vi "MDO-Monitor main_design.vi"() -> ()   [LabVIEW 2012]
uses:
  SubVI/Controls/main_states.ctl
  SubVI/Controls/options.ctl
  SubVI/Controls/Globol_Data_Cluster.ctl
  SubVI/Controls/main_tab.ctl
  SubVI/Controls/process condition.ctl
  SubVI/Controls/MBA_data.ctl
  <vilib>/Utility/miscctls.llb/LVRowAndColumnTypeDef.ctl
  <vilib>/Utility/error.llb/DialogType.ctl
  <vilib>/Utility/file.llb/Write To Spreadsheet File (string).vi
  <vilib>/Analysis/5stat.llb/RMS (DBL).vi
  <vilib>/Analysis/baseanly.llb/Mean (DBL).vi
  <vilib>/Analysis/NI_AALPro.lvlib
  <vilib>/Analysis/NI_AALBase.lvlib
panel:
  out "Sreaming_Execution:State":T1(ring)
  out "Application Directory":path
  out "Max_voltage":dbl
  out "states_history":string
  out "current_state":T2
  out "Main Tab":T3(tab)
  in  "stop":bool
  in  "МДО-Настройщик":bool
  in  "МДО-Монитор":bool
  out "current time":timestamp format="%<%X\n%x>T"
  in  "МДО-Принтер":bool
  in  "МДО-Визуализатор":bool
  in  "Electrolyte composition":string[][](table)=[["KOH", "2"], ["Жидкое стекло", "9"]] caption="Состав электролита"
  in  "Дата проведения процесса":string
  in  "Время проведения процесса":string
  in  "Предмет исследований":string
  in  "Сплав":string
  in  "Очистить все поля":bool
  out "Ti литейные сплавы":string="Ti литейный"
  out "Ti деформируемые сплавы":string="Ti деформ"
  out "Mg литейные сплавы":string="Mg литейный"
  out "Mg деформируемые сплавы":string="Mg деформ"
  out "Al деформируемые сплавы":string="Al деформ"
  out "Al литейные сплавы":string="Al литейный"
  out "Список сплавов":string[][](table)
  in  "MDO_mode":string(combo)="ПОЭП"
  in  "Bath volume":string(combo)="800 л"
  in  "MDO duration":i32
  in  "К процессу":bool
  in  "Пауза":bool
  in  "Принудительный запуск":bool
  in  "Отложенный запуск":bool
  in  "СТОП":bool
  in  "Graph Tab":T4(tab)
  out "Катодный ток, А":cluster{dbl, dbl, dbl}(knob) scale=0.0..40.0
  out "Анодный ток, А":cluster{dbl, dbl, dbl}(knob) scale=0.0..40.0 scale format="%#.1g"
  out "Катодное напряжение, В":cluster{u16, u16, u16}(knob) scale=0.0..200.0
  out "Анодное напряжение, В":cluster{u16, u16, u16}(knob) scale=0.0..800.0
  out "XY Graph":cluster{"all rows":dbl[], "all rows":dbl[]}(graph)
  out "Currency":dbl[](graph)
  out "Voltage":dbl[](graph)
  in  "anod/katod_Form":bool
  out "Формовочный ток":cluster{dbl, dbl, dbl}(graph)
  out "Формовочное напряжение":cluster{u16, u16, u16}(graph)
  out "Process Electrical Parameters":string[][](table)
  out "Bath type":string caption="Ванна"
  out "Electrolyte temperature":dbl(slide) caption="Температура электролита" scale=0.0..60.0
  out "Cooler flow":dbl(knob) caption="Давление воды в системе охлаждения" scale=0.0..3.5 scale format="%#_2g"
  out "Bubbling flow":bool caption="Расход газа в барботере"
  out "Ventilation flow":bool caption="Расход газа в вытяжке"
  in  "ВЫХОД":bool
  in  "НОВЫЙ СБОР":bool
  out "ДАННЫЕ СОХРАНЕНЫ":string="ДАННЫЕ СОХРАНЕНЫ"
  in  "Save_data":bool
  in  "ПРИМЕЧАНИЕ":bool
  in  "ТОК ТОЧНО":u8(slide)=5 max=10 step=1 scale=0.0..10.0
  in  "ТОК ГРУБО":u8(slide)=1 max=2 step=1 scale=0.0..2.0
  in  "ПРЕДЕЛЫ ПО НАПРЯЖ":bool=TRUE
  in  "СТОП - КАДР":bool
  in  "Boolean":bool
  out "ТАЙМЕР Текущий":string
  out "УГАСАНИЕ":string="УГАСАНИЕ"
  out "ДР":string="Д Р"
  out "ИР":string="И Р"
  out "ГАЛЬВ.ЛЮМ.":string="ГАЛЬВ"
  out "МДР":string="МДР"
  out "依商判":string
  out "СТОП":string="СТОП"
  out "ПАУЗА":string="ПАУЗА"
  out "СБОР":string="СБОР"
  out "Готовность":string="ГОТОВ"
  in  "End vizualization":bool
  in  "End print":bool
  in  "Options":T5={"Form_data_log_period"=0, "startup_threshold"=0.0, "Coeff_U"=2.55, "Offset_U"=6.5, "Coeff_I"=42.391, "Offset_I"=77.0, "Save_data_path"=path "", "ADC_frequency"=50000.0, "VISA resource name"="COM1"} caption="Настройки"
  in  "Apply options":bool
  in  "Cancel options":bool
  # "МДО-Монитор"
  # "Мониторинг электрических технологических параметров процесса микродугового оксидирования и обновление базы данных МДО"
  # "МДО-Настройщик"
  # "Настройка параметров \nМДО-Инструментарий"
  # "Пожалуйста, заполните описание эксперимента"
  # "Дата и время проведения процесса"
  # "Цель исследования"
  # "Сплав"
  # "Электролит"
  # "Очистить все поля"
  # "Ванна"
  # "ТИТ"
  # "Длительность"
  # "мин"
  # "ПАНЕЛЬ ЗАПУСКА"
  # "ПУСК СЛЕДЯЩИЙ"
  # "ПУСК ПРИНУДИТ"
  # "ПАУЗА"
  # "СТОП"
  # "АПЛИТУДНЫЙ\nДЕЙСТВУЮЩИЙ\nСРЕДНИЙ"
  # "АПЛИТУДНОЕ\nДЕЙСТВУЮЩЕЕ\nСРЕДНЕЕ"
  # "劳文"
  # "КАТОД"
  # "о"
  # "С"
  # "атм"
  # "ПАНЕЛЬ УПРАВЛЕНИЯ"
  # "ГРУБО"
  # "ТОЧНО"
  # "ПРЕДЕЛЫ"
  # "ПО ТОКУ"
  # "800 /200"
  # "1000 / 250"
  # "ПРЕДЕЛЫ"
  # "ПО НАПРЯЖ"
  # "ПАНЕЛЬ ИНДИКАЦИИ"
  # "Принудительная остановка"
  # "Здесь будет"
  # "Визуализатор"
  # "Визуализация электрических технологических параметров процесса микродугового оксидирования по базе данных МДО"
  # "Здесь будет"
  # "Принтер"
  # "Распечатка графиков электрических параметров процесса МДО (осциллограммы, ВАХи, форовочные кривые) по базе данных МДО"
  # "с"
  # "В"
  # "Настройки АЦП"
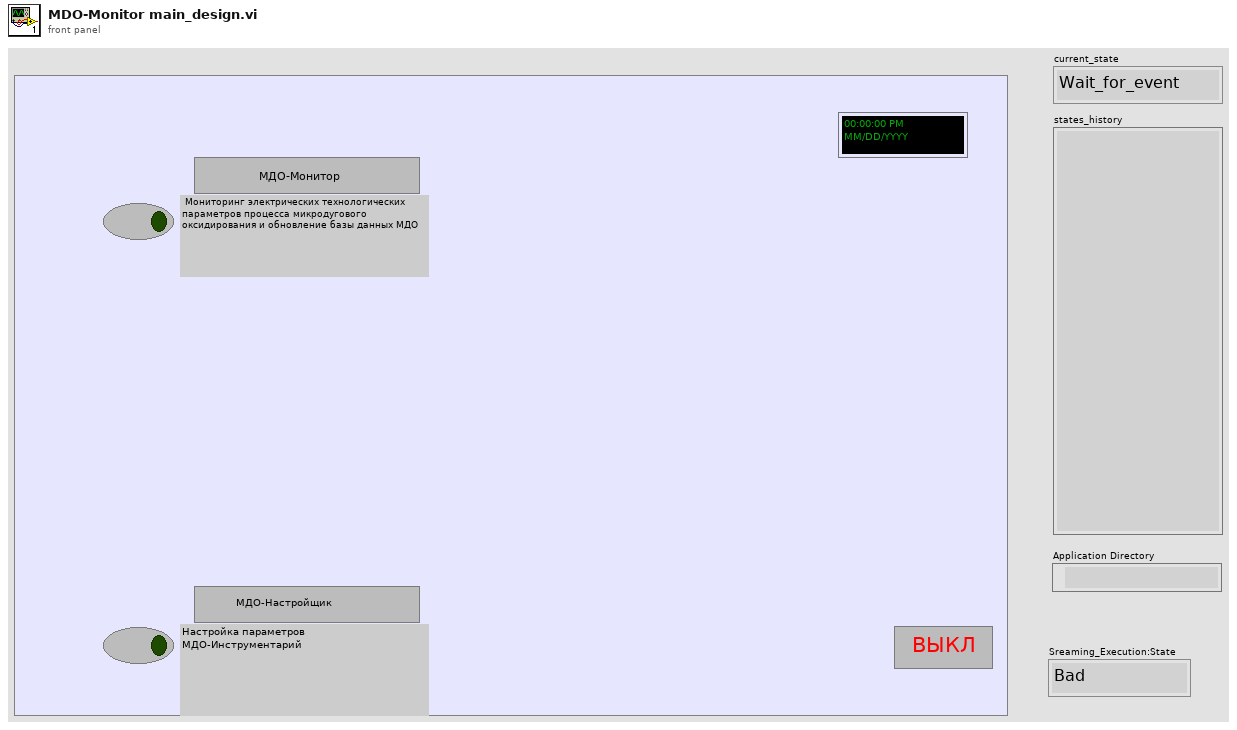
[diagram p1: front panel]
types:
  T1 = enum32{"Bad", "Idle", "Run top level", "Running"}
  T2 = typedef "main_states.ctl" = enum16{"Wait_for_event", "Initialize", "Save_ini", "Save_data", "Streaming_config", "Streaming_open", "Streaming_monitor", "Streaming_stop", "Vizualyze", "Form_data_fetch", "Process_analyze", "Start_data_loging", "Pause_data_loging", "Stop_data_loging", "Reset_data_colection", "Error_handler", "Stop"}
  T3 = enum32{"Выбор", "Описание эксперимента", "Монитор", "Визуализатор", "Принтер", "Настройщик"}
  T4 = enum32{"Осциллограммы/ВАХи", "Формовочные кривые", "Электрические параметры", "Состояние оборудования "}
  T5 = typedef "options.ctl" = cluster{"Form_data_log_period":i32, "startup_threshold":dbl, "Coeff_U":dbl, "Offset_U":dbl, "Coeff_I":dbl, "Offset_I":dbl, "Save_data_path":path, "ADC_frequency":dbl, "VISA resource name":refnum<visa-resource-name>}
  T6 = typedef "Globol_Data_Cluster.ctl" = cluster{"Streaming_enable":bool, "Options":T5, "Ini_file_path":path, "Global_errors":errorcluster, "Main Tab":T7, "Process conditions":T8, "App_directory_path":path, "Data_write_enable":bool, "Process_time":u32, "Current":dbl[], "Voltag":dbl[], "startup_time":u32, "Streaming Refnum":refnum<vi>, "Note Refnum":refnum<vi>, "Note":string, "Modbus spy Refnum":refnum<vi>, "MBA data":T9, "shutdown?":bool, "Oscil_path":path, " Data log path":path}
  T7 = typedef "main_tab.ctl" = enum32{"Выбор", "Описание эксперимента", "Монитор", "Визуализатор", "Принтер", "Настройщик"}
  T8 = typedef "process condition.ctl" = cluster{"Data":string, "Time":string, "Subject":string, "Research target":string, "Material":string, "Electrolyte composition":string[][], "MDO mode":string, "Bath volume":string, "Process duration":i32}
  T9 = typedef "MBA_data.ctl" = cluster{"MBA_ch 1":dbl, "MBA_ch 2":dbl, "MBA_ch 3":dbl, "MBA_ch 4":dbl, "MBA_ch 5":dbl, "MBA_ch 6":dbl, "MBA_ch 7":dbl, "MBA_ch 8":dbl}
  T10 = typedef "LVRowAndColumnTypeDef.ctl" = cluster{"Row":i32, "Column":i32}
  T11 = enum16{"open", "replace", "create", "open or create", "replace or create", "replace or create with confirmation"}
  T12 = enum32{"invalid app kind", "Development System", "Run Time System", "Student Edition", "Embedded LabVIEW", "Evaluation", "Custom"}
  T13 = typedef "DialogType.ctl" = u16
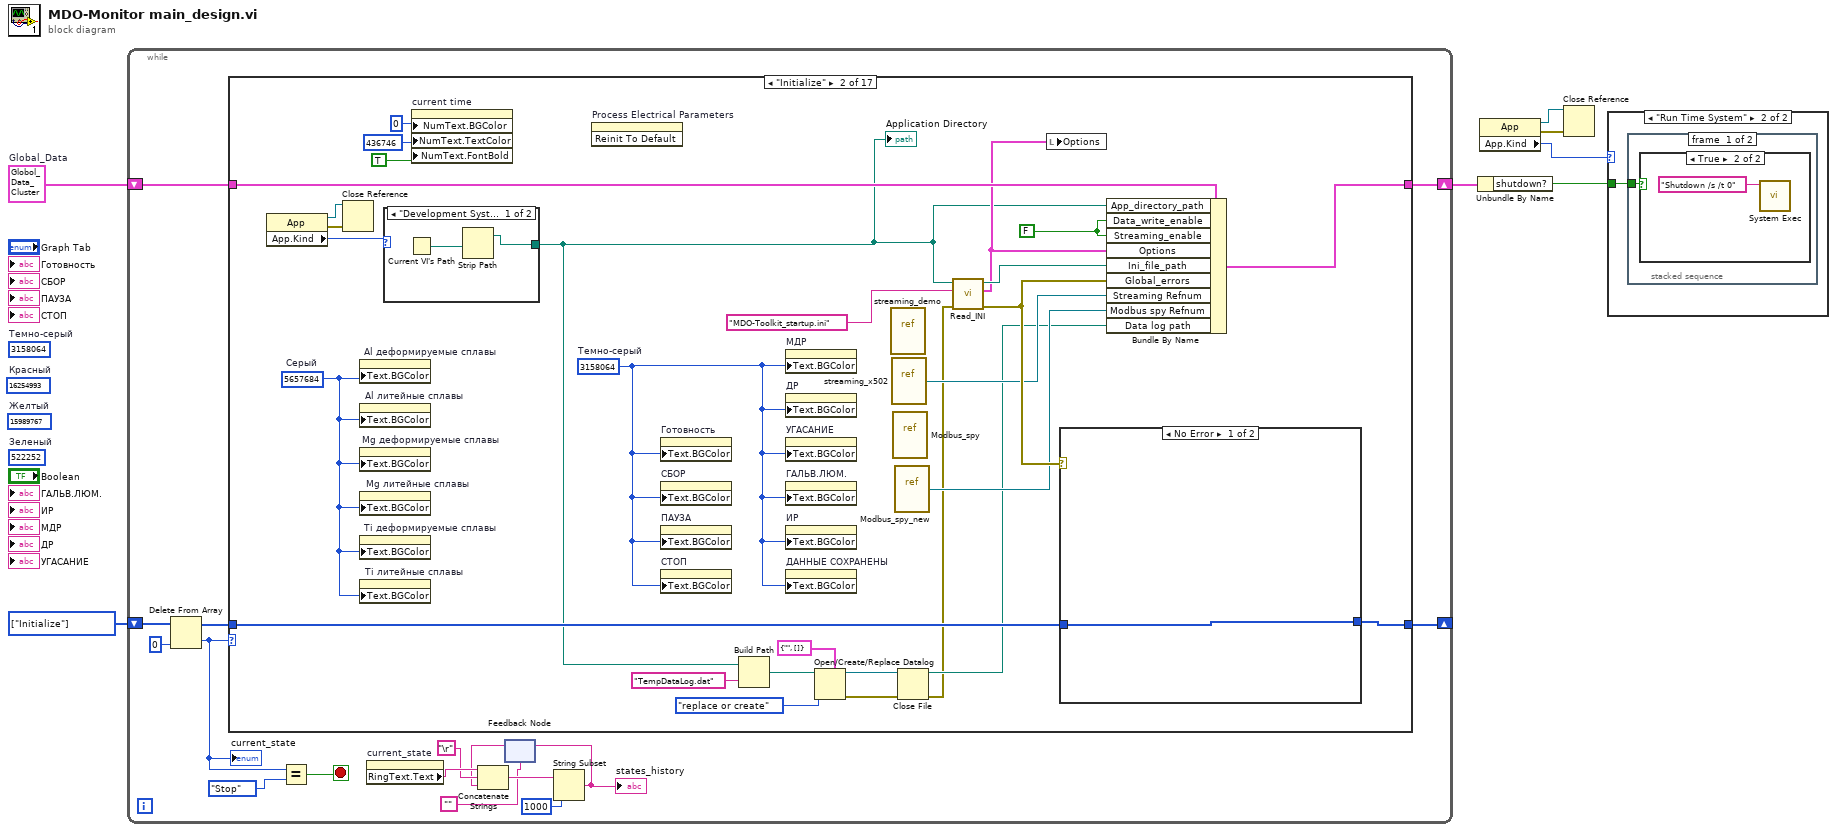
[diagram p0: block diagram]
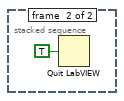
[diagram p4: hidden frame]
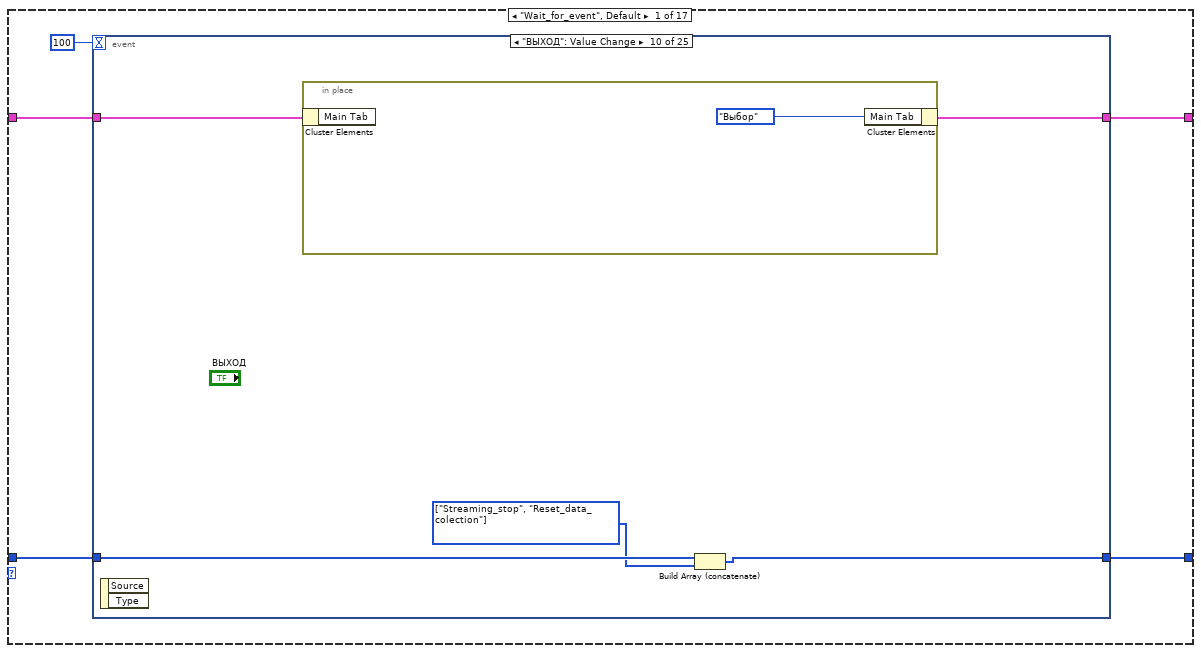
[diagram p5: hidden frame]
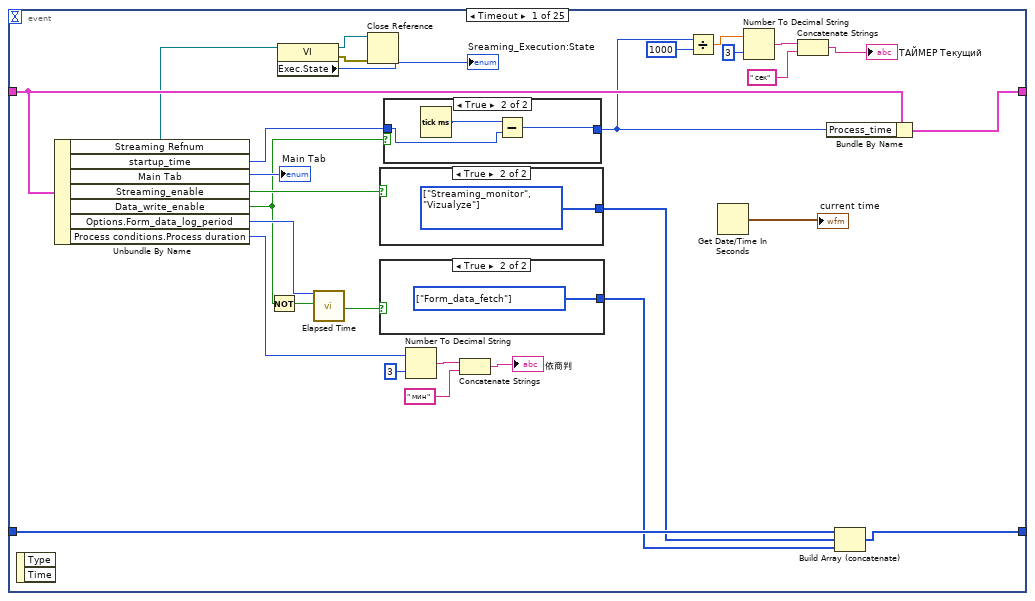
[diagram p6: hidden frame]
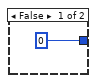
[diagram p7: hidden frame]
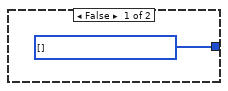
[diagram p8: hidden frame]
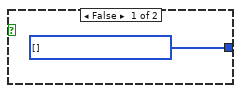
[diagram p9: hidden frame]
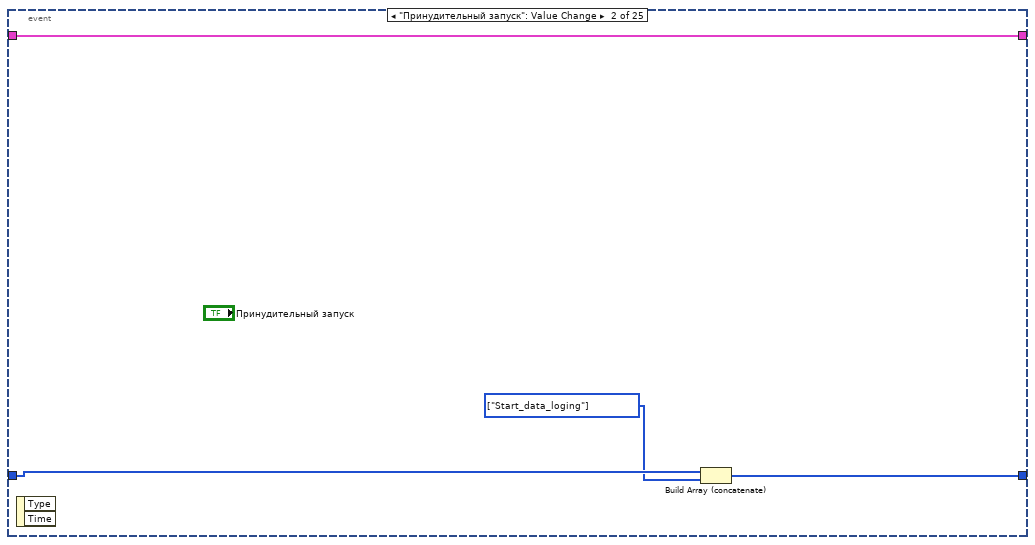
[diagram p10: hidden frame]
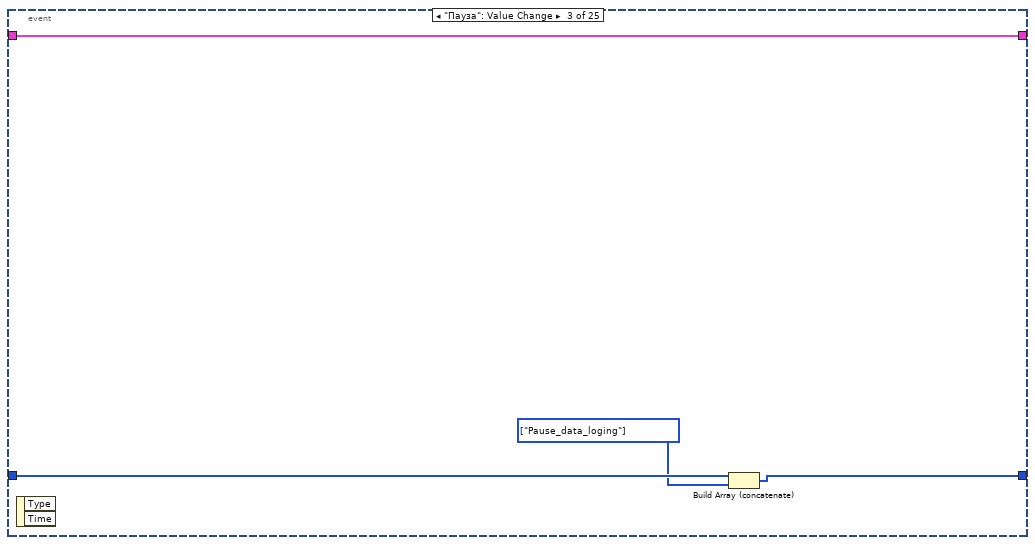
[diagram p11: hidden frame]
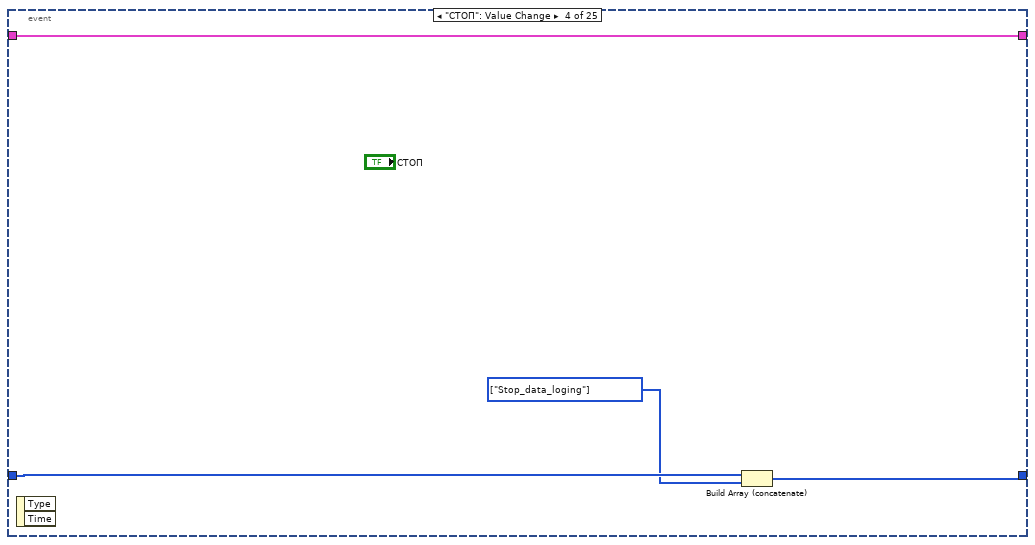
[diagram p12: hidden frame]
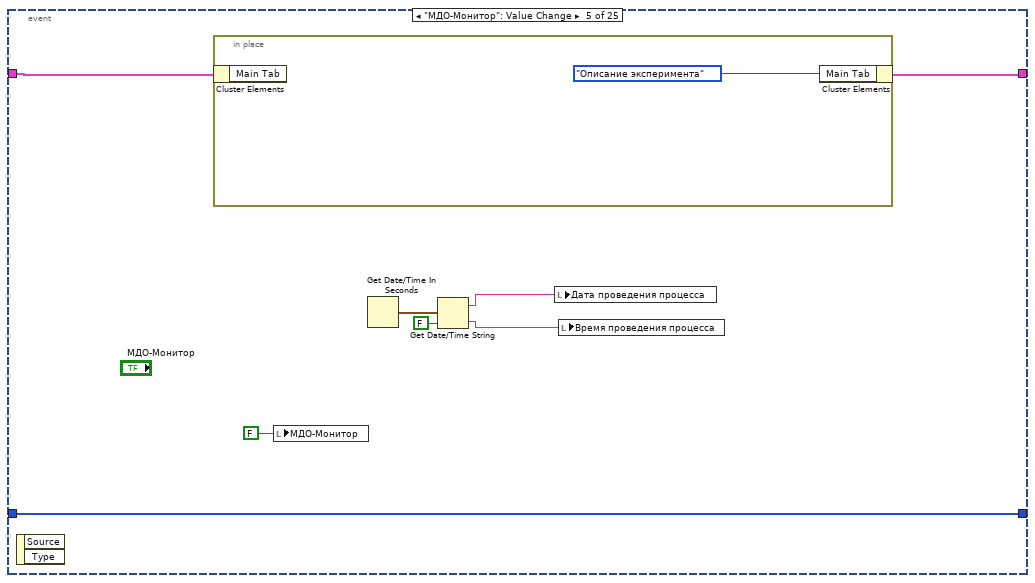
[diagram p13: hidden frame]
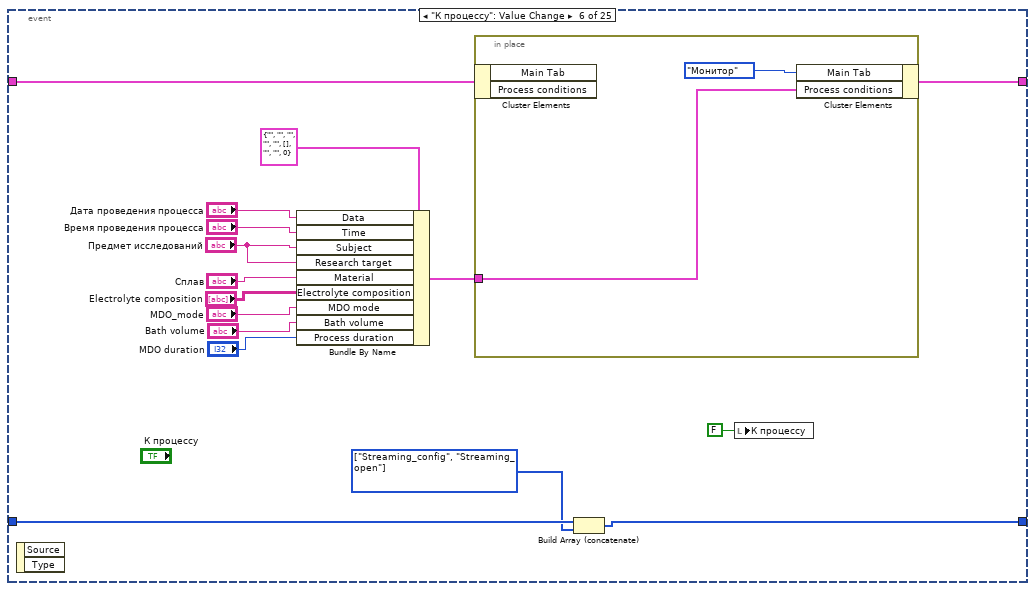
[diagram p14: hidden frame]
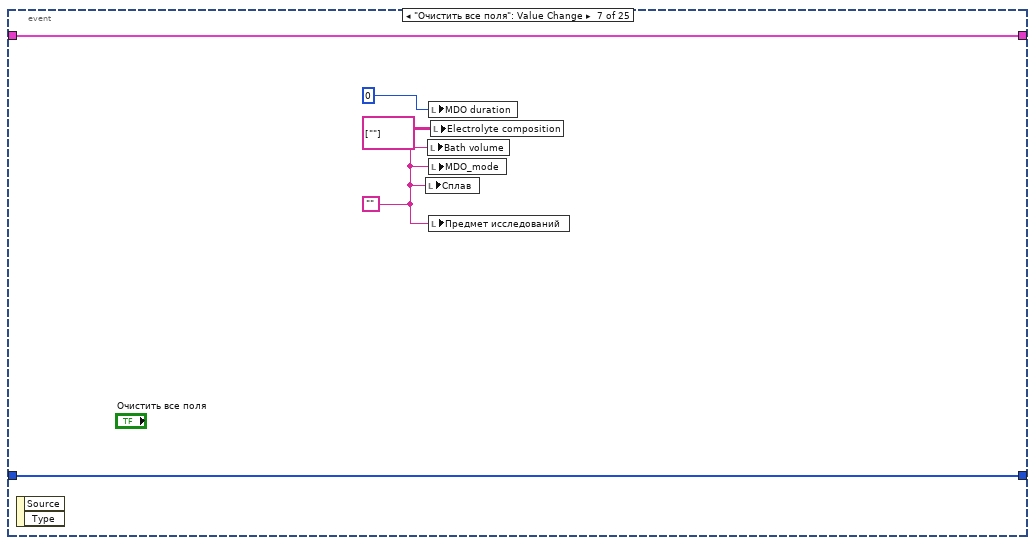
[diagram p15: hidden frame]
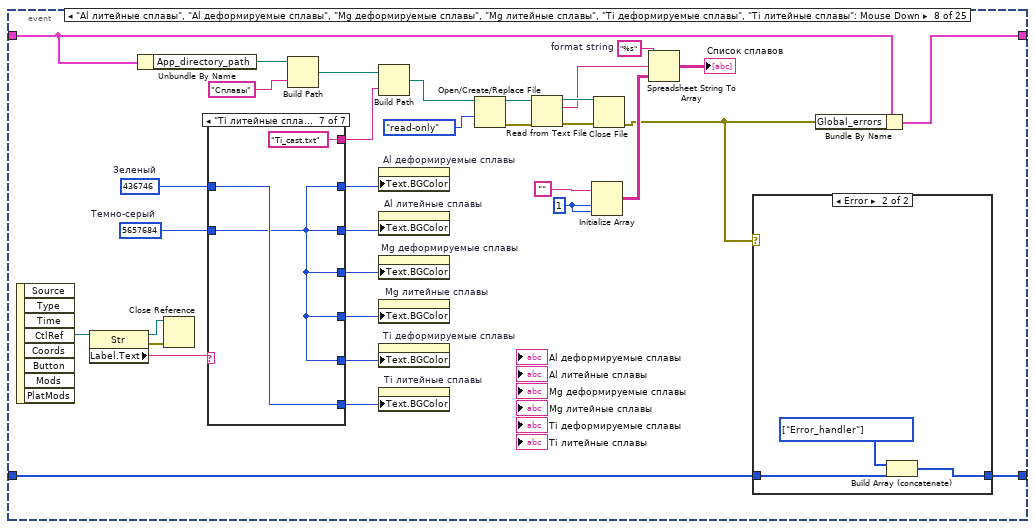
[diagram p16: hidden frame]
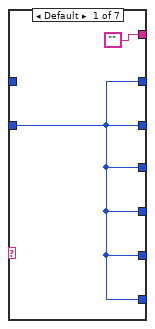
[diagram p18: hidden frame]
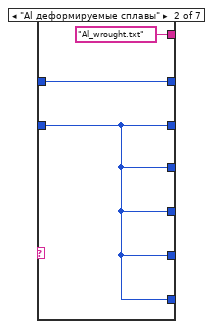
[diagram p19: hidden frame]
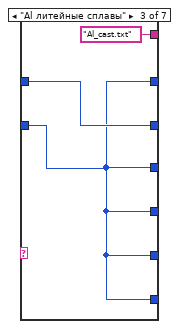
[diagram p20: hidden frame]
diagram:
  (unwired) 522252  # Зеленый
  (unwired) 16254993  # Красный
  (unwired) 3158064  # Темно-серый
  w6 = T6 {"Streaming_enable"=FALSE, "Options"={"Form_data_log_period"=0, "startup_threshold"=0.0, "Coeff_U"=0.0, "Offset_U"=0.0, "Coeff_I"=0.0, "Offset_I"=0.0, "Save_data_path"=path "", "ADC_frequency"=0.0, "VISA resource name"=""}, "Ini_file_path"=path "", "Global_errors"={"status"=FALSE, "code"=0, "source"=""}, "Main Tab"=enum."Выбор", "Process conditions"={"Data"="", "Time"="", "Subject"="", "Research target"="", "Material"="", "Electrolyte composition"=[], "MDO mode"="", "Bath volume"="", "Process duration"=0}, "App_directory_path"=path "", "Data_write_enable"=FALSE, "Process_time"=0, "Current"=[], "Voltag"=[], "startup_time"=0, "Streaming Refnum"=refnum, "Note Refnum"=refnum, "Note"="", "Modbus spy Refnum"=refnum, "MBA data"={"MBA_ch 1"=0.0, "MBA_ch 2"=0.0, "MBA_ch 3"=0.0, "MBA_ch 4"=0.0, "MBA_ch 5"=0.0, "MBA_ch 6"=0.0, "MBA_ch 7"=0.0, "MBA_ch 8"=0.0}, "shutdown?"=FALSE, "Oscil_path"=path "", " Data log path"=path ""}  # Global_Data
  w7 = T2[] [enum."Initialize"] items=["Wait_for_event", "Initialize", "Save_ini", "Save_data", "Streaming_config", "Streaming_open", "Streaming_monitor", "Streaming_stop", "Vizualyze", "Form_data_fetch", "Process_analyze", "Start_data_loging", "Pause_data_loging", "Stop_data_loging", "Reset_data_colection", "Error_handler", "Stop"]
  (unwired) 15989767  # Желтый
  n1 = while {
    shift-right: [w15] -> w5
    shift-left: w6 -> [w16]
    shift-right: [w9] -> _
    shift-left: w7 -> [w10]
    stop <- w23 stop-if-true
    n2 = Delete From Array(array=w10, index=0) -> (deleted portion=w8:T2, array with subset deleted=w14:T2[])  [unwired: 1 in]
    "current_state" <- w8
    n3 = case shown="\"Initialize\"" w8 {
      tunnel: w16 -> [w27 w354 w369 w395 w455 w485 w522 w552 w605 w621 w661 w707 w722 w740 w755 w768 w779]
      tunnel: [w26 w350 w367 w394 w454 w487 w523 w554 w605 w621 w661 w706 w721 w739 w755 w767 w779] -> w15
      tunnel: w14 -> [w25 w353 w365 w393 w457 w488 w525 w549 w588 w659 w680 w708 w720 w738 w764 w766 w780]
      tunnel: [w24 w352 w364 w392 w456 w488 w524 w548 w587 w659 w680 w708 w720 w738 w764 w765 w780] -> w9
      frame "Wait_for_event", Default {
        n4 = event shown="[9] \"ВЫХОД\": Value Change" {
          selector: _ -> [_ _ _ _ _ _ _ _ _ _ _ _ _ _ _ _ _ _ _ _ _ _ _ _ _]
          dyn-events: _ -> [_ _ _ _ _ _ _ _ _ _ _ _ _ _ _ _ _ _ _ _ _ _ _ _ _]
          timeout: 100 -> [_ _ _ _ _ _ _ _ _ _ _ _ _ _ _ _ _ _ _ _ _ _ _ _ _]
          tunnel: w27 -> [w49 w70 w74 w78 w85 w103 w110 w117 w182 w187 w192 w196 w237 w243 w250 w263 w266 w270 w275 w280 w284 w297 w301 w306 w317]
          tunnel: [w48 w70 w74 w78 w84 w102 w110 w116 w182 w186 w192 w195 w237 w243 w250 w263 w265 w269 w274 w279 w283 w296 w300 w306 w316] -> w26
          tunnel: w25 -> [w53 w69 w73 w77 w86 w92 w109 w114 w181 w185 w191 w197 w240 w244 w249 w262 w267 w271 w276 w278 w287 w295 w299 w304 w319]
          tunnel: [w50 w67 w71 w76 w86 w91 w109 w113 w181 w184 w190 w197 w239 w244 w249 w262 w267 w271 w276 w278 w286 w294 w299 w303 w318] -> w24
          event Timeout {
            n5 = event-data() -> ()  [unwired: 1 in, 2 out]
            n6 = Unbundle By Name(w49) -> ("Streaming Refnum"=w32:refnum<vi>, "startup_time"=w41:u32, "Main Tab"=→"Main Tab":T7, "Streaming_enable"=w57:bool, "Data_write_enable"=w47:bool, "Options.Form_data_log_period"=w55:i32, "Process conditions.Process duration"=w46:i32)
            n7 = Not(x=w47) -> (.not. x?=w56:bool)
            n8 = property class="VI"(reference=w32) -> (reference out=w30:refnum<vi>, error out=w31:errorcluster, "Exec.State"=→"Sreaming_Execution:State":T1)  [unwired: 1 in]
            n9 = call "Elapsed Time"("Time Target (s)"=w55, "Reset"=w56) -> ("Time has Elapsed"=w54:bool)  [unwired: 10 in, 7 out]
            n10 = Close Reference(reference=w30, error in (no error)=w31) -> ()  [unwired: 1 out]
            n11 = case shown="True" w57 {
              tunnel: [w65 w66] -> w52
              frame False {
                w65 = T2[] [] items=["Wait_for_event", "Initialize", "Save_ini", "Save_data", "Streaming_config", "Streaming_open", "Streaming_monitor", "Streaming_stop", "Vizualyze", "Form_data_fetch", "Process_analyze", "Start_data_loging", "Pause_data_loging", "Stop_data_loging", "Reset_data_colection", "Error_handler", "Stop"] ("array")
              }
              frame True {
                w66 = T2[] [enum."Streaming_monitor", enum."Vizualyze"] items=["Wait_for_event", "Initialize", "Save_ini", "Save_data", "Streaming_config", "Streaming_open", "Streaming_monitor", "Streaming_stop", "Vizualyze", "Form_data_fetch", "Process_analyze", "Start_data_loging", "Pause_data_loging", "Stop_data_loging", "Reset_data_colection", "Error_handler", "Stop"] ("array")
              }
            }
            n12 = case shown="True" w54 {
              tunnel: [w63 w64] -> w51
              frame False {
                w63 = T2[] [] items=["Wait_for_event", "Initialize", "Save_ini", "Save_data", "Streaming_config", "Streaming_open", "Streaming_monitor", "Streaming_stop", "Vizualyze", "Form_data_fetch", "Process_analyze", "Start_data_loging", "Pause_data_loging", "Stop_data_loging", "Reset_data_colection", "Error_handler", "Stop"] ("array")
              }
              frame True {
                w64 = T2[] [enum."Form_data_fetch"] items=["Wait_for_event", "Initialize", "Save_ini", "Save_data", "Streaming_config", "Streaming_open", "Streaming_monitor", "Streaming_stop", "Vizualyze", "Form_data_fetch", "Process_analyze", "Start_data_loging", "Pause_data_loging", "Stop_data_loging", "Reset_data_colection", "Error_handler", "Stop"] ("array")
              }
            }
            n13 = case shown="True" w47 {
              tunnel: w41 -> [_ w62]
              tunnel: [u32 0 w60] -> w39
              frame False {
              }
              frame True {
                n14 = Tick Count (ms)() -> (millisecond timer value=w61:u32)
                n15 = Subtract(x=w61, y=w62) -> (x-y=w60:u32)
              }
            }
            n16 = Number To Decimal String(number=w46, width (-)=i16 3) -> (decimal integer string=w44:string)
            n17 = Concatenate Strings(w44, " мин" ("string")) -> (→"依商判":string)
            n18 = Divide(x=w39, y=u32 1000) -> (x/y=w34:dbl)
            n19 = Get Date/Time In Seconds() -> (seconds since 1Jan1904=→"current time":timestamp)
            n20 = Number To Decimal String(number=w34, width (-)=i16 3) -> (decimal integer string=w36:string)
            n21 = Concatenate Strings(w36, " сек" ("string")) -> (→"ТАЙМЕР Текущий":string)
            n22 = Bundle By Name(cluster=w49, "Process_time"=w39) -> (w48:T6)
            n23 = Build Array (concatenate)(w53, w52, w51) -> (w50:T2[])
          }
          event "Принудительный запуск": Value Change {
            w68 = T2[] [enum."Start_data_loging"] items=["Wait_for_event", "Initialize", "Save_ini", "Save_data", "Streaming_config", "Streaming_open", "Streaming_monitor", "Streaming_stop", "Vizualyze", "Form_data_fetch", "Process_analyze", "Start_data_loging", "Pause_data_loging", "Stop_data_loging", "Reset_data_colection", "Error_handler", "Stop"] ("array")
            n24 = event-data() -> ()  [unwired: 1 in, 2 out]
            n25 = Build Array (concatenate)(w69, w68) -> (w67:T2[])
          }
          event "Пауза": Value Change {
            w72 = T2[] [enum."Pause_data_loging"] items=["Wait_for_event", "Initialize", "Save_ini", "Save_data", "Streaming_config", "Streaming_open", "Streaming_monitor", "Streaming_stop", "Vizualyze", "Form_data_fetch", "Process_analyze", "Start_data_loging", "Pause_data_loging", "Stop_data_loging", "Reset_data_colection", "Error_handler", "Stop"] ("array")
            n26 = event-data() -> ()  [unwired: 1 in, 2 out]
            n27 = Build Array (concatenate)(w73, w72) -> (w71:T2[])
          }
          event "СТОП": Value Change {
            w75 = T2[] [enum."Stop_data_loging"] items=["Wait_for_event", "Initialize", "Save_ini", "Save_data", "Streaming_config", "Streaming_open", "Streaming_monitor", "Streaming_stop", "Vizualyze", "Form_data_fetch", "Process_analyze", "Start_data_loging", "Pause_data_loging", "Stop_data_loging", "Reset_data_colection", "Error_handler", "Stop"] ("array")
            n28 = event-data() -> ()  [unwired: 1 in, 2 out]
            n29 = Build Array (concatenate)(w77, w75) -> (w76:T2[])
          }
          event "МДО-Монитор": Value Change {
            n30 = event-data() -> ()  [unwired: 1 in, 2 out]
            n31 = in-place {
              n32 = in-place-cluster #1(w85) -> ()  [unwired: 1 out]
              n33 = in-place-cluster #1("Main Tab"=main_tab."Описание эксперимента") -> (w84:T6)
            }
            n34 = local write "МДО-Монитор"(FALSE ("МДО-Монитор")) -> ()
            n35 = Get Date/Time In Seconds() -> (seconds since 1Jan1904=w83:timestamp)
            n36 = Get Date/Time String(seconds (now)=w83, want seconds? (F)=FALSE) -> (date string=w80:string, time string=w81:string)  [unwired: 1 in]
            n37 = local write "Дата проведения процесса"(w80) -> ()
            n38 = local write "Время проведения процесса"(w81) -> ()
          }
          event "К процессу": Value Change {
            w90 = T2[] [enum."Streaming_config", enum."Streaming_open"] items=["Wait_for_event", "Initialize", "Save_ini", "Save_data", "Streaming_config", "Streaming_open", "Streaming_monitor", "Streaming_stop", "Vizualyze", "Form_data_fetch", "Process_analyze", "Start_data_loging", "Pause_data_loging", "Stop_data_loging", "Reset_data_colection", "Error_handler", "Stop"] ("array")
            n39 = event-data() -> ()  [unwired: 1 in, 2 out]
            n40 = Bundle By Name(cluster=T8 {"Data"="", "Time"="", "Subject"="", "Research target"="", "Material"="", "Electrolyte composition"=[], "MDO mode"="", "Bath volume"="", "Process duration"=0} ("Process conditions"), "Data"="Дата проведения процесса", "Time"="Время проведения процесса", "Subject"="Предмет исследований", "Research target"="Предмет исследований", "Material"="Сплав", "Electrolyte composition"="Electrolyte composition", "MDO mode"="MDO_mode", "Bath volume"="Bath volume", "Process duration"="MDO duration") -> (w100:T8)
            n41 = in-place {
              in-place-border: w100 -> [w104]
              n42 = in-place-cluster #2(w103) -> ()  [unwired: 2 out]
              n43 = in-place-cluster #2("Main Tab"=main_tab."Монитор", "Process conditions"=w104) -> (w102:T6)
            }
            n44 = Build Array (concatenate)(w92, w90) -> (w91:T2[])
            n45 = local write "К процессу"(FALSE ("К процессу")) -> ()
          }
          event "Очистить все поля": Value Change {
            w106 = ""
            n46 = event-data() -> ()  [unwired: 1 in, 2 out]
            n47 = local write "Сплав"(w106) -> ()
            n48 = local write "Bath volume"(w106) -> ()
            n49 = local write "MDO duration"(u16 0 ("MDO duration")) -> ()
            n50 = local write "MDO_mode"(w106) -> ()
            n51 = local write "Предмет исследований"(w106) -> ()
            n52 = local write "Electrolyte composition"(string[][] [[""]] ("Electrolyte composition")) -> ()
          }
          event "Al литейные сплавы", "Al деформируемые сплавы", "Mg деформируемые сплавы", "Mg литейные сплавы", "Ti деформируемые сплавы", "Ti литейные сплавы": Mouse Down {
            w131 = 1
            w129 = "%s"  # format string
            w140 = 436746  # Зеленый
            w141 = 5657684  # Темно-серый
            n53 = event-data() -> ("CtlRef"=w143:refnum<vi>)  [unwired: 1 in, 7 out]
            n54 = property class="Str"(reference=w143) -> (reference out=w111:refnum<vi>, error out=w112:errorcluster, "Label.Text"=w142:string)  [unwired: 1 in]
            n55 = Unbundle By Name(w117) -> ("App_directory_path"=w122:path)
            n56 = Close Reference(reference=w111, error in (no error)=w112) -> ()  [unwired: 1 out]
            n57 = case shown="\"Ti литейные сплавы\"" w142 {
              tunnel: w141 -> [w149 w151 w154 w157 w160 w163 w166]
              tunnel: w140 -> [_ w152 w155 w158 w161 w164 w167]
              tunnel: [w149 w152 w154 w157 w160 w163 w166] -> w139
              tunnel: [w149 w151 w155 w157 w160 w163 w166] -> w138
              tunnel: [w149 w151 w154 w158 w160 w163 w166] -> w137
              tunnel: [w149 w151 w154 w157 w161 w163 w166] -> w136
              tunnel: [w149 w151 w154 w157 w160 w164 w166] -> w135
              tunnel: [w149 w151 w154 w157 w160 w163 w167] -> w134
              tunnel: ["" "Al_wrought.txt" "Al_cast.txt" "Mg_wrought.txt" "Mg_cast.txt" "Ti_wrought.txt" "Ti_cast.txt"] -> w119
              frame Default {
              }
              frame "Al деформируемые сплавы" {
              }
              frame "Al литейные сплавы" {
              }
              frame "Mg деформируемые сплавы" {
              }
              frame "Mg литейные сплавы" {
              }
              frame "Ti деформируемые сплавы" {
              }
              frame "Ti литейные сплавы" {
              }
            }
            n58 = Build Path(base path=w122, name or relative path="Сплавы") -> (appended path=w120:path)
            n59 = Build Path(base path=w120, name or relative path=w119) -> (appended path=w118:path)
            n60 = property on="Al деформируемые сплавы" class="Str"("Text.BGColor"=w139) -> ()  [unwired: 2 in, 2 out]
            n61 = property on="Al литейные сплавы" class="Str"("Text.BGColor"=w138) -> ()  [unwired: 2 in, 2 out]
            n62 = property on="Mg деформируемые сплавы" class="Str"("Text.BGColor"=w137) -> ()  [unwired: 2 in, 2 out]
            n63 = property on="Mg литейные сплавы" class="Str"("Text.BGColor"=w136) -> ()  [unwired: 2 in, 2 out]
            n64 = property on="Ti деформируемые сплавы" class="Str"("Text.BGColor"=w135) -> ()  [unwired: 2 in, 2 out]
            n65 = property on="Ti литейные сплавы" class="Str"("Text.BGColor"=w134) -> ()  [unwired: 2 in, 2 out]
            n66 = Open/Create/Replace File(file path (use dialog)=w118, access (0:read/write)=enum16{"read/write", "read-only", "write-only"}."read-only") -> (refnum out=w127:refnum<file>, error out=w128:errorcluster)  [unwired: 4 in, 1 out]
            n67 = Read from Text File(file (use dialog)=w127, error in=w128) -> (refnum out=w125:refnum<file>, text=w124:string, error out=w126:errorcluster)  [unwired: 2 in, 1 out]
            n68 = Initialize Array("", w131, w131) -> (w132:string[][])
            n69 = Close File(refnum=w125, error in=w126) -> (error out=w115:errorcluster)  [unwired: 1 out]
            n70 = Spreadsheet String To Array(format string=w129, spreadsheet string=w124, array type (2D Dbl)=w132) -> (array=→"Список сплавов":string[][])  [unwired: 1 in]
            n71 = case shown="Error" w115 {
              tunnel: w114 -> [w144 w147]
              tunnel: [w144 w146] -> w113
              frame No Error {
              }
              frame Error {
                w145 = T2[] [enum."Error_handler"] items=["Wait_for_event", "Initialize", "Save_ini", "Save_data", "Streaming_config", "Streaming_open", "Streaming_monitor", "Streaming_stop", "Vizualyze", "Form_data_fetch", "Process_analyze", "Start_data_loging", "Pause_data_loging", "Stop_data_loging", "Reset_data_colection", "Error_handler", "Stop"] ("array")
                n72 = Build Array (concatenate)(w145, w147) -> (w146:T2[])
              }
            }
            n73 = Bundle By Name(cluster=w117, "Global_errors"=w115) -> (w116:T6)
          }
          event "Список сплавов": Mouse Down {
            n74 = event-data() -> ("CtlRef"=w180:refnum<vi>)  [unwired: 1 in, 7 out]
            n75 = property class="Tbl (strict)"(reference=w180) -> (reference out=w179:refnum<vi>, error out=w173:errorcluster, "EditPos"=w176:T10)  [unwired: 1 in]
            n76 = property class="Tbl (strict)"(reference=w179, error in=w173) -> (reference out=w172:refnum<vi>, error out=w171:errorcluster, "Value"=w178:string[][])
            n77 = Unbundle By Name(w176) -> ("Row"=w175:i32, "Column"=w174:i32)
            n78 = Index Array(array=w178, index (row)=w175, index (col)=w174) -> (element=w177:string)
            n79 = local write "Сплав"(w177) -> ()
            n80 = property class="Tbl (strict)"(reference=w172, error in=w171, "EditPos"=T10 {"Row"=-1, "Column"=-1} ("Edit Position")) -> (reference out=w169:refnum<vi>, error out=w170:errorcluster)
            n81 = Close Reference(reference=w169, error in (no error)=w170) -> ()  [unwired: 1 out]
          }
          event "ВЫХОД": Value Change {
            w183 = T2[] [enum."Streaming_stop", enum."Reset_data_colection"] items=["Wait_for_event", "Initialize", "Save_ini", "Save_data", "Streaming_config", "Streaming_open", "Streaming_monitor", "Streaming_stop", "Vizualyze", "Form_data_fetch", "Process_analyze", "Start_data_loging", "Pause_data_loging", "Stop_data_loging", "Reset_data_colection", "Error_handler", "Stop"] ("array")
            n82 = event-data() -> ()  [unwired: 1 in, 2 out]
            n83 = in-place {
              n84 = in-place-cluster #3(w187) -> ()  [unwired: 1 out]
              n85 = in-place-cluster #3("Main Tab"=main_tab."Выбор") -> (w186:T6)
            }
            n86 = Build Array (concatenate)(w185, w183) -> (w184:T2[])
          }
          event "НОВЫЙ СБОР": Value Change {
            w189 = T2[] [enum."Reset_data_colection"] items=["Wait_for_event", "Initialize", "Save_ini", "Save_data", "Streaming_config", "Streaming_open", "Streaming_monitor", "Streaming_stop", "Vizualyze", "Form_data_fetch", "Process_analyze", "Start_data_loging", "Pause_data_loging", "Stop_data_loging", "Reset_data_colection", "Error_handler", "Stop"] ("array")
            n87 = event-data() -> ()  [unwired: 1 in, 2 out]
            n88 = Build Array (concatenate)(w191, w189) -> (w190:T2[])
          }
          event "ПРИМЕЧАНИЕ": Value Change {
            n89 = event-data() -> ()  [unwired: 1 in, 2 out]
            n90 = vi-ref "note.vi"() -> (w193:refnum<vi>)
            n91 = case shown="False" "ПРИМЕЧАНИЕ" {
              tunnel: w196 -> [w207 w233]
              tunnel: [w206 w233] -> w195
              tunnel: w193 -> [w202 w225]
              frame False {
                n92 = call "Read_indicator_in_stream.vi"("Required_indicatorl_name"="Canceled?", "reference"=w202) -> ("error out"=w199:errorcluster, "Value"=w204:variant, "reference out"=w200:refnum<vi>)  [unwired: 7 in]
                n93 = Variant To Data(error in=w199, type=TRUE, Variant=w204) -> (data=w201:bool, error out=w198:errorcluster)
                n94 = case shown="False" w201 {
                  tunnel: w207 -> [w211 w224]
                  tunnel: [w210 w224] -> w206
                  tunnel: w200 -> [w209 _]
                  tunnel: w198 -> [w208 _]
                  frame False {
                    n95 = in-place {
                      in-place-border: w209 -> [w215]
                      in-place-border: w208 -> [w214]
                      w222 = "\r"
                      n96 = in-place-cluster #4(w211) -> ("Process_time"=w213:u32, "Note"=w216:string)
                      n97 = call "Read_indicator_in_stream.vi"("error in (no error)"=w214, "Required_indicatorl_name"="out", "reference"=w215) -> ("error out"=w219:errorcluster, "Value"=w220:variant)  [unwired: 6 in, 1 out]
                      n98 = Variant To Data(error in=w219, type="" ("string"), Variant=w220) -> (data=w218:string)  [unwired: 1 out]
                      n99 = call "process time convertion.vi"("process_time"=w213) -> ("out"=w212:string)
                      n100 = Concatenate Strings(w216, w212, w218, w222, w222) -> (w223:string)
                      n101 = in-place-cluster #4("Process_time"=w213, "Note"=w223) -> (w210:T6)
                    }
                  }
                  frame True {
                  }
                }
              }
              frame True {
                n102 = control-ref of="ПРИМЕЧАНИЕ"() -> (w226:refnum<vi>)
                n103 = call "Write_control_in_stream.vi"("Value"=w226, "Required_control_name"="Ctl Refnum", "reference"=w225) -> ("reference out"=w228:refnum<vi>)  [unwired: 8 in]
                n104 = invoke class="VI" method="FP.Open"(reference=w228, "Activate"=TRUE ("Activate?")) -> (reference out=w231:refnum<vi>, error out=w229:errorcluster)  [unwired: 3 in, 3 out]
                n105 = invoke class="VI" method="Run VI"(reference=w231, error in=w229, "Wait until done"=FALSE ("Wait Until Done")) -> (reference out=w232:refnum<vi>, error out=w235:errorcluster)  [unwired: 2 in, 3 out]
                n106 = Close Reference(reference=w232, error in (no error)=w235) -> ()  [unwired: 1 out]
              }
            }
          }
          event "Save_data": Value Change {
            w238 = T2[] [enum."Save_data"] items=["Wait_for_event", "Initialize", "Save_ini", "Save_data", "Streaming_config", "Streaming_open", "Streaming_monitor", "Streaming_stop", "Vizualyze", "Form_data_fetch", "Process_analyze", "Start_data_loging", "Pause_data_loging", "Stop_data_loging", "Reset_data_colection", "Error_handler", "Stop"] ("array")
            n107 = event-data() -> ()  [unwired: 1 in, 2 out]
            n108 = local write "Save_data"(FALSE ("Save_data")) -> ()
            n109 = Build Array (concatenate)(w240, w238) -> (w239:T2[])
          }
          event "СТОП - КАДР": Value Change {
            n110 = event-data() -> ()  [unwired: 1 in, 2 out]
            n111 = local write "СТОП - КАДР"(FALSE ("СТОП - КАДР")) -> ()
            n112 = One Button Dialog(message="Эта функция пока не работает") -> ()  [unwired: 1 in, 1 out]
          }
          event "ПРЕДЕЛЫ ПО НАПРЯЖ": Value Change {
            n113 = event-data() -> ()  [unwired: 1 in, 2 out]
            n114 = case shown="True" "ПРЕДЕЛЫ ПО НАПРЯЖ" {
              tunnel: [1000.0 ("Y Scale.Range:Maximum") 800.0 ("Y Scale.Range:Maximum")] -> w247
              tunnel: [-250.0 ("Y Scale.Range:Minimum") -200.0 ("Y Scale.Range:Minimum")] -> w245
              frame False {
              }
              frame True {
              }
            }
            n115 = Negate(x=w245) -> (-x=w246:dbl)
            n116 = property on="Voltage" class="WFGraph (strict)"("YScale.Maximum"=w247, "YScale.Minimum"=w245) -> ()  [unwired: 2 in, 2 out]
            n117 = property on="XY Graph" class="XYGraph (strict)"("YScale.Maximum"=w247, "YScale.Minimum"=w245) -> ()  [unwired: 2 in, 2 out]
            n118 = property on="Катодное напряжение, В" class="Knob (strict)"("Scale.Maximum"=w246) -> ()  [unwired: 2 in, 2 out]
            n119 = property on="Анодное напряжение, В" class="Knob (strict)"("Scale.Maximum"=w247) -> ()  [unwired: 2 in, 2 out]
          }
          event "ТОК ГРУБО", "ТОК ТОЧНО": Value Change {
            n120 = event-data() -> ()  [unwired: 1 in, 2 out]
            n121 = Increment(x="ТОК ГРУБО") -> (x+1=w257:u8)
            n122 = Multiply(x=10.0, y=w257) -> (x*y=w260:dbl)
            n123 = Add(x=w260, y="ТОК ТОЧНО") -> (x+y=w255:dbl)
            n124 = Negate(x=w255) -> (-x=w256:dbl)
            n125 = property on="Катодный ток, А" class="Knob (strict)"("Scale.Maximum"=w255) -> ()  [unwired: 2 in, 2 out]
            n126 = property on="Currency" class="WFGraph (strict)"("YScale.Maximum"=w255, "YScale.Minimum"=w256) -> ()  [unwired: 2 in, 2 out]
            n127 = property on="Анодный ток, А" class="Knob (strict)"("Scale.Maximum"=w255) -> ()  [unwired: 2 in, 2 out]
            n128 = property on="XY Graph" class="XYGraph (strict)"("XScale.Maximum"=w255, "XScale.Minimum"=w256) -> ()  [unwired: 2 in, 2 out]
          }
          event "МДО-Визуализатор": Value Change {
            n129 = event-data() -> ()  [unwired: 1 in, 2 out]
            n130 = in-place {
              n131 = in-place-cluster #5(w266) -> ()  [unwired: 1 out]
              n132 = in-place-cluster #5("Main Tab"=main_tab."Визуализатор") -> (w265:T6)
            }
            n133 = local write "МДО-Визуализатор"(FALSE ("МДО-Визуализатор")) -> ()
          }
          event "End vizualization": Value Change {
            n134 = event-data() -> ()  [unwired: 1 in, 2 out]
            n135 = in-place {
              n136 = in-place-cluster #6(w270) -> ()  [unwired: 1 out]
              n137 = in-place-cluster #6("Main Tab"=main_tab."Выбор") -> (w269:T6)
            }
          }
          event "МДО-Принтер": Value Change {
            n138 = event-data() -> ()  [unwired: 1 in, 2 out]
            n139 = in-place {
              n140 = in-place-cluster #7(w275) -> ()  [unwired: 1 out]
              n141 = in-place-cluster #7("Main Tab"=main_tab."Принтер") -> (w274:T6)
            }
            n142 = local write "МДО-Принтер"(FALSE ("МДО-Принтер")) -> ()
          }
          event "End print": Value Change {
            n143 = event-data() -> ()  [unwired: 1 in, 2 out]
            n144 = in-place {
              n145 = in-place-cluster #8(w280) -> ()  [unwired: 1 out]
              n146 = in-place-cluster #8("Main Tab"=main_tab."Выбор") -> (w279:T6)
            }
          }
          event "МДО-Настройщик": Value Change {
            w285 = T2[] [] items=["Wait_for_event", "Initialize", "Save_ini", "Save_data", "Streaming_config", "Streaming_open", "Streaming_monitor", "Streaming_stop", "Vizualyze", "Form_data_fetch", "Process_analyze", "Start_data_loging", "Pause_data_loging", "Stop_data_loging", "Reset_data_colection", "Error_handler", "Stop"] ("array")
            n147 = event-data() -> ()  [unwired: 1 in, 2 out]
            n148 = in-place {
              n149 = in-place-cluster #9(w284) -> ()  [unwired: 1 out]
              n150 = in-place-cluster #9("Main Tab"=main_tab."Настройщик") -> (w283:T6)
            }
            n151 = local write "МДО-Настройщик"(FALSE ("МДО-Настройщик")) -> ()
            n152 = Build Array (concatenate)(w287, w285) -> (w286:T2[])
          }
          event "Apply options", "Cancel options": Value Change {
            w289 = FALSE ("Cancel options")
            w291 = T2[] [] items=["Wait_for_event", "Initialize", "Save_ini", "Save_data", "Streaming_config", "Streaming_open", "Streaming_monitor", "Streaming_stop", "Vizualyze", "Form_data_fetch", "Process_analyze", "Start_data_loging", "Pause_data_loging", "Stop_data_loging", "Reset_data_colection", "Error_handler", "Stop"] ("array")
            w292 = T2[] [enum."Save_ini"] items=["Wait_for_event", "Initialize", "Save_ini", "Save_data", "Streaming_config", "Streaming_open", "Streaming_monitor", "Streaming_stop", "Vizualyze", "Form_data_fetch", "Process_analyze", "Start_data_loging", "Pause_data_loging", "Stop_data_loging", "Reset_data_colection", "Error_handler", "Stop"] ("array")
            n153 = event-data() -> ()  [unwired: 1 in, 3 out]
            n154 = in-place {
              n155 = in-place-cluster #10(w297) -> ()  [unwired: 1 out]
              n156 = in-place-cluster #10("Main Tab"=main_tab."Выбор") -> (w296:T6)
            }
            n157 = Select(t=w292, s="Apply options", f=w291) -> (s? t:f=w290:T2[])
            n158 = local write "Cancel options"(w289) -> ()
            n159 = local write "Apply options"(w289) -> ()
            n160 = Build Array (concatenate)(w295, w290) -> (w294:T2[])
          }
          event Value Change {
            n161 = event-data() -> ()  [unwired: 1 in, 6 out]
            n162 = in-place {
              n163 = in-place-cluster #11(w301) -> ()  [unwired: 1 out]
              n164 = in-place-cluster #11("Options"="Options") -> (w300:T6)
            }
          }
          event Panel Close? {
            n165 = event-data() -> ()  [unwired: 1 in, 2 out]
            n166 = Two Button Dialog(message="Вы действительно хотите закрыть программу?", 1:"Нет" ("F button name (\"Cancel\")"), 2:"Да" ("T button name (\"OK\")")) -> (T button?=w305:bool)
            n167 = case shown="True" w305 {
              tunnel: w304 -> [w311 w314]
              tunnel: [w311 w313] -> w303
              frame False {
              }
              frame True {
                w312 = T2[] [enum."Streaming_stop", enum."Stop"] items=["Wait_for_event", "Initialize", "Save_ini", "Save_data", "Streaming_config", "Streaming_open", "Streaming_monitor", "Streaming_stop", "Vizualyze", "Form_data_fetch", "Process_analyze", "Start_data_loging", "Pause_data_loging", "Stop_data_loging", "Reset_data_colection", "Error_handler", "Stop"] ("array")
                n168 = Build Array (concatenate)(w314, w312) -> (w313:T2[])
              }
            }
            n169 = event-data("Discard?"=TRUE) -> ()  [unwired: 1 in, 1 out]
          }
          event "stop": Value Change {
            n170 = event-data() -> ()  [unwired: 1 in, 2 out]
            n171 = Two Button Dialog(message="Вы действительно хотите выключить систему мониторинга?", 1:"Нет" ("F button name (\"Cancel\")"), 2:"Да" ("T button name (\"OK\")")) -> (T button?=w315:bool)
            n172 = case shown="True" w315 {
              tunnel: w319 -> [w324 w327]
              tunnel: [w324 w326] -> w318
              frame False {
              }
              frame True {
                w325 = T2[] [enum."Streaming_stop", enum."Stop"] items=["Wait_for_event", "Initialize", "Save_ini", "Save_data", "Streaming_config", "Streaming_open", "Streaming_monitor", "Streaming_stop", "Vizualyze", "Form_data_fetch", "Process_analyze", "Start_data_loging", "Pause_data_loging", "Stop_data_loging", "Reset_data_colection", "Error_handler", "Stop"] ("array")
                n173 = Build Array (concatenate)(w327, w325) -> (w326:T2[])
              }
            }
            n174 = in-place {
              in-place-border: w315 -> [w323]
              n175 = in-place-cluster #12(w317) -> ()  [unwired: 1 out]
              n176 = in-place-cluster #12("shutdown?"=w323) -> (w316:T6)
            }
          }
        }
      }
      frame "Initialize" {
        w341 = 3158064  # Темно-серый
        w342 = 5657684  # Cерый
        w340 = FALSE ("Streaming_enable")
        n177 = property class="App"() -> (reference out=w344:refnum<vi>, error out=w345:errorcluster, "App.Kind"=w355:T12)  [unwired: 2 in]
        n178 = Close Reference(reference=w344, error in (no error)=w345) -> ()  [unwired: 1 out]
        n179 = property on="Al деформируемые сплавы" class="Str"("Text.BGColor"=w342) -> ()  [unwired: 2 in, 2 out]
        n180 = property on="Al литейные сплавы" class="Str"("Text.BGColor"=w342) -> ()  [unwired: 2 in, 2 out]
        n181 = property on="Mg деформируемые сплавы" class="Str"("Text.BGColor"=w342) -> ()  [unwired: 2 in, 2 out]
        n182 = property on="Mg литейные сплавы" class="Str"("Text.BGColor"=w342) -> ()  [unwired: 2 in, 2 out]
        n183 = property on="Ti деформируемые сплавы" class="Str"("Text.BGColor"=w342) -> ()  [unwired: 2 in, 2 out]
        n184 = property on="Ti литейные сплавы" class="Str"("Text.BGColor"=w342) -> ()  [unwired: 2 in, 2 out]
        n185 = case shown="\"Development System\", Default" w355 {
          tunnel: [w360 w362] -> w328
          frame "Development System", Default {
            n186 = Current VI's Path() -> (path=w361:path)
            n187 = Strip Path(path=w361) -> (stripped path=w360:path)  [unwired: 1 out]
          }
          frame "Run Time System" {
            n188 = call <vilib>:"Application Directory.vi"() -> ("Application Directory"=w362:path)
          }
        }
        "Application Directory" <- w328
        n189 = property on="current time" class="AbsTime (strict)"("NumText.BGColor"=u32 0 ("Numeric Text.Text Colors:BG Color"), "NumText.TextColor"=u32 436746 ("Numeric Text.Text Colors:Text Color"), "NumText.FontBold"=TRUE ("Numeric Text.Font:Bold")) -> ()  [unwired: 2 in, 2 out]
        n190 = invoke on="Process Electrical Parameters" class="Tbl (strict)" method="Reinit To Default"() -> ()  [unwired: 3 in, 3 out]
        n191 = property on="Готовность" class="Str"("Text.BGColor"=w341) -> ()  [unwired: 2 in, 2 out]
        n192 = property on="СБОР" class="Str"("Text.BGColor"=w341) -> ()  [unwired: 2 in, 2 out]
        n193 = property on="ПАУЗА" class="Str"("Text.BGColor"=w341) -> ()  [unwired: 2 in, 2 out]
        n194 = property on="СТОП" class="Str"("Text.BGColor"=w341) -> ()  [unwired: 2 in, 2 out]
        n195 = Build Path(base path=w328, name or relative path="TempDataLog.dat") -> (appended path=w334:path)
        n196 = property on="МДР" class="Str"("Text.BGColor"=w341) -> ()  [unwired: 2 in, 2 out]
        n197 = property on="ДР" class="Str"("Text.BGColor"=w341) -> ()  [unwired: 2 in, 2 out]
        n198 = property on="УГАСАНИЕ" class="Str"("Text.BGColor"=w341) -> ()  [unwired: 2 in, 2 out]
        n199 = property on="ГАЛЬВ.ЛЮМ." class="Str"("Text.BGColor"=w341) -> ()  [unwired: 2 in, 2 out]
        n200 = property on="ИР" class="Str"("Text.BGColor"=w341) -> ()  [unwired: 2 in, 2 out]
        n201 = property on="ДАННЫЕ СОХРАНЕНЫ" class="Str"("Text.BGColor"=w341) -> ()  [unwired: 2 in, 2 out]
        n202 = Open/Create/Replace Datalog(5:cluster{string, "empty array":sgl[]} {"", "empty array"=[]}, 10:T11."replace or create" ("operation (0:open)"), 11:w334) -> (0:w332:errorcluster, 3:w331:refnum<k1>)  [unwired: 1 in, 3 out]
        n203 = vi-ref "streaming_demo.vi"() -> ()  [unwired: 1 out]
        n204 = vi-ref "streaming_x502.vi"() -> (w338:refnum<vi>)
        n205 = vi-ref "Modbus_spy.vi"() -> ()  [unwired: 1 out]
        n206 = vi-ref "Modbus_spy_new.vi"() -> (w337:refnum<vi>)
        n207 = Close File(refnum=w331, error in=w332) -> (path=w330:path, error out=w329:errorcluster)
        n208 = call "Read_INI.vi"("error in (no error)"=w329, "INI_file_name"="MDO-Toolkit_startup.ini", "App_directory"=w328) -> ("error out"=w351:errorcluster, "Options"=w339:T5, "file path"=w349:path)  [unwired: 6 in]
        n209 = local write "Options"(w339) -> ()
        n210 = case shown="No Error" w351 {
          tunnel: w353 -> [w356 w358]
          tunnel: [w356 w359] -> w352
          frame No Error {
          }
          frame Error {
            w357 = T2[] [enum."Error_handler"] items=["Wait_for_event", "Initialize", "Save_ini", "Save_data", "Streaming_config", "Streaming_open", "Streaming_monitor", "Streaming_stop", "Vizualyze", "Form_data_fetch", "Process_analyze", "Start_data_loging", "Pause_data_loging", "Stop_data_loging", "Reset_data_colection", "Error_handler", "Stop"] ("array")
            n211 = Build Array (concatenate)(w357, w358) -> (w359:T2[])
          }
        }
        n212 = Bundle By Name(cluster=w354, "App_directory_path"=w328, "Data_write_enable"=w340, "Streaming_enable"=w340, "Options"=w339, "Ini_file_path"=w349, "Global_errors"=w351, "Streaming Refnum"=w338, "Modbus spy Refnum"=w337, "Data log path"=w330) -> (w350:T6)
      }
      frame "Save_ini" {
        n213 = Unbundle By Name(w369) -> ("Ini_file_path"=w370:path, "Options"=w363:T5)
        n214 = call "Write_INI.vi"("Options"=w363, "Ini_file_path"=w370) -> ("error out"=w366:errorcluster, "Ini_file_path_out"=w368:path)  [unwired: 8 in]
        n215 = case shown="No Error" w366 {
          tunnel: w365 -> [w371 w372]
          tunnel: [w371 w374] -> w364
          frame No Error {
          }
          frame Error {
            w373 = T2[] [enum."Error_handler"] items=["Wait_for_event", "Initialize", "Save_ini", "Save_data", "Streaming_config", "Streaming_open", "Streaming_monitor", "Streaming_stop", "Vizualyze", "Form_data_fetch", "Process_analyze", "Start_data_loging", "Pause_data_loging", "Stop_data_loging", "Reset_data_colection", "Error_handler", "Stop"] ("array")
            n216 = Build Array (concatenate)(w373, w372) -> (w374:T2[])
          }
        }
        n217 = Bundle By Name(cluster=w369, "Ini_file_path"=w368, "Global_errors"=w366) -> (w367:T6)
      }
      frame "Save_data" {
        w399 = "\r"
        n218 = Unbundle By Name(w395) -> ("Options.Save_data_path"=w389:path, "Process conditions.Data"=w397:string, "Process conditions.Time"=w434:string, "Process conditions.Subject"=w384:string, "Process conditions.Research target"=w432:string, "Process conditions.Material"=w430:string, "Process conditions.Electrolyte composition"=w421:string[][], "Process conditions.MDO mode"=w428:string, "Process conditions.Bath volume"=w426:string, "Process conditions.Process duration"=w424:i32, "Note"=w390:string, "Data log path"=w378:path)
        n219 = property on="Process Electrical Parameters" class="Tbl (strict)"() -> ("Column Headers[]"=w401:string[], "Value"=w402:string[][])  [unwired: 2 in, 2 out]
        n220 = Build Array (concatenate)(w401, w402) -> (w400:string[][])
        n221 = call <vilib>:"Space Constant.vi"() -> ("String"=w396:string)
        n222 = Concatenate Strings("Дата и время проведения:  " ("string"), w397, w396, w434) -> (w418:string)
        n223 = Concatenate Strings("Предмет исследования:  " ("string"), w384) -> (w417:string)
        n224 = Concatenate Strings("Цель исследования:  " ("string"), w432) -> (w416:string)
        n225 = Concatenate Strings("Сплав:  " ("string"), w430) -> (w415:string)
        n226 = Concatenate Strings("Режим обработки:  " ("string"), w428) -> (w413:string)
        n227 = Concatenate Strings("Ванна:   " ("string"), w426) -> (w412:string)
        n228 = Number To Decimal String(number=w424) -> (decimal integer string=w423:string)  [unwired: 1 in]
        n229 = Array To Spreadsheet String(delimiter (Tab)="\t", array=w400, 3:"%3d" ("format string")) -> (spreadsheet string=w391:string)
        n230 = Concatenate Strings("Длительность процесса, мин:   " ("string"), w423) -> (w411:string)
        n231 = Array To Spreadsheet String(delimiter (Tab)="\t", array=w421, 3:"%3d" ("format string")) -> (spreadsheet string=w419:string)
        n232 = call "File Dialog"("start path"=w389, "default name"=w384) -> ("selected path"=w383:path, "cancelled"=w385:bool, "error out"=w386:errorcluster)  [unwired: 10 in, 1 out]
        n233 = Concatenate Strings("Состав электролита:  " ("string"), "\r", w419) -> (w414:string)
        n234 = Build Array(w418, w417, w416, w415, w414, w413, w412, w411, w399, w399, w390, w391) -> (w410:string[])
        n235 = Strip Path(path=w383) -> (stripped path=w380:path, name=w382:string)
        n236 = call "Read_Temp_Data_Log.vi"("DataLogPath"=w378) -> ("error out"=w375:errorcluster, "Data"=w376:string[][])  [unwired: 9 in]
        n237 = Array To Spreadsheet String(delimiter (Tab)="\r", array=w410, 3:"%3d" ("format string")) -> (spreadsheet string=w387:string)
        n238 = Concatenate Strings(w382, "Oscill.txt" ("string")) -> (w379:string)
        n239 = call <vilib>:"Simple Error Handler.vi"("error in (no error)"=w375) -> ()  [unwired: 4 in, 5 out]
        n240 = case shown="False" w385 {
          tunnel: [w439 errorcluster {"status"=FALSE, "code"=0, "source"=""} ("error out")] -> w388
          tunnel: w383 -> [w438 _]
          tunnel: w387 -> [w437 _]
          tunnel: w386 -> [w436 _]
          frame False {
            w435 = 522252  # Зеленый
            n241 = Write to Text File(file (use dialog)=w438, text=w437, error in=w436) -> (refnum out=w440:refnum<file>, error out=w441:errorcluster)  [unwired: 1 in, 1 out]
            n242 = property on="ДАННЫЕ СОХРАНЕНЫ" class="Str"("Text.BGColor"=w435) -> ()  [unwired: 2 in, 2 out]
            n243 = Close File(refnum=w440, error in=w441) -> (error out=w439:errorcluster)  [unwired: 1 out]
          }
          frame True {
          }
        }
        n244 = Build Path(base path=w380, name or relative path=w379) -> (appended path=w377:path)
        n245 = call-poly <vilib>:"Write To Spreadsheet File.vi"("2D data"=w376, "file path (dialog if empty)"=w377) -> ()  [unwired: 6 in, 1 out]
        n246 = case shown="No Error" w388 {
          tunnel: w393 -> [w443 w445]
          tunnel: [w443 w444] -> w392
          frame No Error {
          }
          frame Error {
            w446 = T2[] [enum."Error_handler"] items=["Wait_for_event", "Initialize", "Save_ini", "Save_data", "Streaming_config", "Streaming_open", "Streaming_monitor", "Streaming_stop", "Vizualyze", "Form_data_fetch", "Process_analyze", "Start_data_loging", "Pause_data_loging", "Stop_data_loging", "Reset_data_colection", "Error_handler", "Stop"] ("array")
            n247 = Build Array (concatenate)(w446, w445) -> (w444:T2[])
          }
        }
        n248 = Bundle By Name(cluster=w395, "Global_errors"=w388) -> (w394:T6)
      }
      frame "Streaming_config" {
        n249 = Unbundle By Name(w455) -> ("Streaming Refnum"=w470:refnum<vi>, "Options.Coeff_U"=w467:dbl, "Options.Offset_U"=w465:dbl, "Options.Coeff_I"=w464:dbl, "Options.Offset_I"=w461:dbl, "Modbus spy Refnum"=w453:refnum<vi>, "Options.VISA resource name"=w451:refnum<visa-resource-name>)
        n250 = call "Write_control_in_stream.vi"("Value"=w467, "Required_control_name"="Coeff_U", "reference"=w470) -> ("reference out"=w466:refnum<vi>)  [unwired: 8 in]
        n251 = call "Write_control_in_stream.vi"("Value"=w451, "Required_control_name"="VISA resource name", "reference"=w453) -> ("reference out"=w450:refnum<vi>)  [unwired: 8 in]
        n252 = call "Write_control_in_stream.vi"("Value"=w465, "Required_control_name"="Offset_U", "reference"=w466) -> ("reference out"=w463:refnum<vi>)  [unwired: 8 in]
        n253 = Close Reference(reference=w450) -> (error out=w448:errorcluster)  [unwired: 1 in]
        n254 = call "Write_control_in_stream.vi"("Value"=w464, "Required_control_name"="Coeff_I", "reference"=w463) -> ("reference out"=w460:refnum<vi>)  [unwired: 8 in]
        n255 = call "Write_control_in_stream.vi"("Value"=w461, "Required_control_name"="Offset_I", "reference"=w460) -> ("reference out"=w458:refnum<vi>)  [unwired: 8 in]
        n256 = Close Reference(reference=w458) -> (error out=w449:errorcluster)  [unwired: 1 in]
        n257 = Merge Errors(w449, w448) -> (w447:errorcluster)
        n258 = case shown="Error" w447 {
          tunnel: w457 -> [w471 w474]
          tunnel: [w471 w473] -> w456
          frame No Error {
          }
          frame Error {
            w472 = T2[] [enum."Error_handler"] items=["Wait_for_event", "Initialize", "Save_ini", "Save_data", "Streaming_config", "Streaming_open", "Streaming_monitor", "Streaming_stop", "Vizualyze", "Form_data_fetch", "Process_analyze", "Start_data_loging", "Pause_data_loging", "Stop_data_loging", "Reset_data_colection", "Error_handler", "Stop"] ("array")
            n259 = Build Array (concatenate)(w472, w474) -> (w473:T2[])
          }
        }
        n260 = Bundle By Name(cluster=w455, "Global_errors"=w447) -> (w454:T6)
      }
      frame "Streaming_open" {
        n261 = Unbundle By Name(w485) -> ("Streaming Refnum"=w481:refnum<vi>, "Modbus spy Refnum"=w475:refnum<vi>)
        n262 = invoke class="VI" method="Run VI"(reference=w481, "Wait until done"=FALSE ("Wait Until Done")) -> (reference out=w482:refnum<vi>, error out=w483:errorcluster)  [unwired: 3 in, 3 out]
        n263 = invoke class="VI" method="Run VI"(reference=w475, "Wait until done"=FALSE ("Wait Until Done")) -> (reference out=w478:refnum<vi>, error out=w477:errorcluster)  [unwired: 3 in, 3 out]
        n264 = Close Reference(reference=w482, error in (no error)=w483) -> (error out=w480:errorcluster)
        n265 = Close Reference(reference=w478, error in (no error)=w477) -> (error out=w479:errorcluster)
        n266 = call <vilib>:"Clear Errors.vi"("error in (no error)"=w480) -> ()  [unwired: 6 in, 1 out]
        n267 = call <vilib>:"Clear Errors.vi"("error in (no error)"=w479) -> ()  [unwired: 6 in, 1 out]
        n268 = Bundle By Name(cluster=w485, "Streaming_enable"=TRUE) -> (w487:T6)
      }
      frame "Streaming_monitor" {
        w508 = dbl[] []
        w493 = "error out" ("Required_indicatorl_name")
        n269 = Unbundle By Name(w522) -> ("Streaming Refnum"=w521:refnum<vi>, "Modbus spy Refnum"=w504:refnum<vi>)
        n270 = call "Read_indicator_in_stream.vi"("Required_indicatorl_name"="Напряжение", "reference"=w521) -> ("error out"=w500:errorcluster, "Value"=w509:variant, "reference out"=w520:refnum<vi>)  [unwired: 7 in]
        n271 = call "Read_indicator_in_stream.vi"("Required_indicatorl_name"="MBA data", "reference"=w504) -> ("error out"=w495:errorcluster, "Value"=w502:variant, "reference out"=w494:refnum<vi>)  [unwired: 7 in]
        n272 = Variant To Data(error in=w500, type=w508, Variant=w509) -> (data=w515:dbl[], error out=w499:errorcluster)
        n273 = call "Read_indicator_in_stream.vi"("error in (no error)"=w499, "Required_indicatorl_name"="Ток", "reference"=w520) -> ("error out"=w498:errorcluster, "Value"=w516:variant, "reference out"=w519:refnum<vi>)  [unwired: 6 in]
        n274 = Variant To Data(error in=w495, type=T9 {"MBA_ch 1"=0.0, "MBA_ch 2"=0.0, "MBA_ch 3"=0.0, "MBA_ch 4"=0.0, "MBA_ch 5"=0.0, "MBA_ch 6"=0.0, "MBA_ch 7"=0.0, "MBA_ch 8"=0.0} ("MBA data"), Variant=w502) -> (data=w503:T9, error out=w491:errorcluster)
        n275 = disable-structure shown="Enabled" {
          disable-tunnel: w494 -> [w534 w536]
          disable-tunnel: w493 -> [w533 _]
          disable-tunnel: w491 -> [w528 _]
          disable-tunnel: [w527 w535] -> w490
          disable-tunnel: [w526 w535] -> w489
          frame Disabled {
            n276 = call "Read_indicator_in_stream.vi"("Required_indicatorl_name"=w533, "reference"=w534) -> ("error out"=w532:errorcluster, "Value"=w529:variant, "reference out"=w530:refnum<vi>)  [unwired: 7 in]
            n277 = Close Reference(reference=w530, error in (no error)=w532) -> (error out=w531:errorcluster)
            n278 = Variant To Data(error in=w531, type=w528, Variant=w529) -> (data=w527:errorcluster, error out=w526:errorcluster)
          }
          frame Enabled {
            n279 = Close Reference(reference=w536) -> (error out=w535:errorcluster)  [unwired: 1 in]
          }
        }
        n280 = Variant To Data(error in=w498, type=w508, Variant=w516) -> (data=w514:dbl[], error out=w497:errorcluster)
        n281 = call "Read_indicator_in_stream.vi"("error in (no error)"=w497, "Required_indicatorl_name"=w493, "reference"=w519) -> ("error out"=w496:errorcluster, "Value"=w513:variant, "reference out"=w512:refnum<vi>)  [unwired: 6 in]
        n282 = Close Reference(reference=w512, error in (no error)=w496) -> (error out=w492:errorcluster)
        n283 = Variant To Data(error in=w492, type=w492, Variant=w513) -> (data=w510:errorcluster, error out=w511:errorcluster)
        n284 = Merge Errors(w510, w511, w491, w490, w489) -> (w506:errorcluster)
        n285 = Not(x=w506) -> (.not. x?=w507:bool)
        n286 = case shown="Error" w506 {
          tunnel: w525 -> [w537 w540]
          tunnel: [w537 w539] -> w524
          frame No Error {
          }
          frame Error {
            w538 = T2[] [enum."Error_handler"] items=["Wait_for_event", "Initialize", "Save_ini", "Save_data", "Streaming_config", "Streaming_open", "Streaming_monitor", "Streaming_stop", "Vizualyze", "Form_data_fetch", "Process_analyze", "Start_data_loging", "Pause_data_loging", "Stop_data_loging", "Reset_data_colection", "Error_handler", "Stop"] ("array")
            n287 = Build Array (concatenate)(w540, w538) -> (w539:T2[])
          }
        }
        n288 = Bundle By Name(cluster=w522, "Voltag"=w515, "Current"=w514, "Global_errors"=w506, "Streaming_enable"=w507, "MBA data"=w503) -> (w523:T6)
      }
      frame "Streaming_stop" {
        w545 = TRUE
        w546 = "Стоп" ("Required_control_name")
        w553 = FALSE ("Streaming_enable")
        n289 = Unbundle By Name(w552) -> ("Streaming Refnum"=w551:refnum<vi>, "Modbus spy Refnum"=w544:refnum<vi>)
        n290 = call "Write_control_in_stream.vi"("Value"=w545, "Required_control_name"=w546, "reference"=w551) -> ("reference out"=w550:refnum<vi>)  [unwired: 8 in]
        n291 = call "Write_control_in_stream.vi"("Value"=w545, "Required_control_name"=w546, "reference"=w544) -> ("reference out"=w547:refnum<vi>)  [unwired: 8 in]
        n292 = Close Reference(reference=w547) -> (error out=w542:errorcluster)  [unwired: 1 in]
        n293 = Close Reference(reference=w550) -> (error out=w543:errorcluster)  [unwired: 1 in]
        n294 = Merge Errors(w543, w542) -> (w541:errorcluster)
        n295 = case shown="Error" w541 {
          tunnel: w549 -> [w555 w557]
          tunnel: [w555 w556] -> w548
          frame No Error {
          }
          frame Error {
            w558 = T2[] [enum."Error_handler"] items=["Wait_for_event", "Initialize", "Save_ini", "Save_data", "Streaming_config", "Streaming_open", "Streaming_monitor", "Streaming_stop", "Vizualyze", "Form_data_fetch", "Process_analyze", "Start_data_loging", "Pause_data_loging", "Stop_data_loging", "Reset_data_colection", "Error_handler", "Stop"] ("array")
            n296 = Build Array (concatenate)(w558, w557) -> (w556:T2[])
          }
        }
        n297 = Bundle By Name(cluster=w552, "Streaming_enable"=w553, "Data_write_enable"=w553, "Global_errors"=w541) -> (w554:T6)
      }
      frame "Vizualyze" {
        # "Амплитудное\nДействующее \nСреднее"
        n298 = Unbundle By Name(w605) -> ("Process conditions.Bath volume"=w570:string, "MBA data"=w571:T9, "Voltag"=w585:dbl[], "Current"=w584:dbl[], "Data_write_enable"=w593:bool, "Options.startup_threshold"=w594:dbl)
        "Voltage" <- w585
        "Currency" <- w584
        "Bath type" <- w570
        n299 = Unbundle By Name(w571) -> ("MBA_ch 3"=w567:dbl, "MBA_ch 7"=w566:dbl, "MBA_ch 6"=w563:dbl)
        n300 = call "trigger.vi"() -> ()  [unwired: 5 in, 1 out]
        n301 = Bundle("Current"=w584, "Voltag"=w585) -> (→"XY Graph":cluster{"Current":dbl[], "Voltag":dbl[]})  [unwired: 1 in]
        n302 = call "A-K separation.vi"("Input wave"=w585) -> ("Katod wave (inverted)"=w583:waveform(dbl), "Anod wave"=w582:waveform(dbl))  [unwired: 3 in]
        n303 = Greater?(x=w567, y=10.0) -> (0:→"Ventilation flow":bool)
        n304 = Greater?(x=w566, y=80.0) -> (0:→"Bubbling flow":bool)
        n305 = Multiply(x=w563, y=1.0) -> (x*y=→"Cooler flow":dbl)
        n306 = Unbundle By Name(w582) -> ("Y"=w581:dbl[])
        n307 = Unbundle By Name(w583) -> ("Y"=w579:dbl[])
        n308 = Array Max & Min(array=w581) -> (max value=w580:dbl)  [unwired: 3 out]
        n309 = call-poly <vilib>:"RMS.vi"("X"=w581) -> ("rms value"=w606:dbl)  [unwired: 1 out]
        n310 = call-poly <vilib>:"Mean.vi"("X"=w581) -> ("mean"=w604:dbl)  [unwired: 1 out]
        n311 = Array Max & Min(array=w579) -> (max value=w578:dbl)  [unwired: 3 out]
        n312 = call-poly <vilib>:"RMS.vi"("X"=w579) -> ("rms value"=w602:dbl)  [unwired: 1 out]
        n313 = call-poly <vilib>:"Mean.vi"("X"=w579) -> ("mean"=w601:dbl)  [unwired: 1 out]
        n314 = Not(x=w593) -> (.not. x?=w591:bool)
        n315 = Greater?(x=w580, y=w594) -> (0:w592:bool)
        n316 = Bundle(w580, "rms value"=w606, "mean"=w604) -> (→"Анодное напряжение, В":cluster{dbl, "rms value":dbl, "mean":dbl})  [unwired: 1 in]
        n317 = Bundle(w578, "rms value"=w602, "mean"=w601) -> (→"Катодное напряжение, В":cluster{dbl, "rms value":dbl, "mean":dbl})  [unwired: 1 in]
        n318 = Compound Arithmetic op=AND(w592, w591, "Отложенный запуск") -> (w589:bool)
        n319 = case shown="False" w589 {
          tunnel: [w617 w618] -> w586
          frame False {
            w617 = T2[] [] items=["Wait_for_event", "Initialize", "Save_ini", "Save_data", "Streaming_config", "Streaming_open", "Streaming_monitor", "Streaming_stop", "Vizualyze", "Form_data_fetch", "Process_analyze", "Start_data_loging", "Pause_data_loging", "Stop_data_loging", "Reset_data_colection", "Error_handler", "Stop"] ("array")
          }
          frame True {
            w618 = T2[] [enum."Start_data_loging"] items=["Wait_for_event", "Initialize", "Save_ini", "Save_data", "Streaming_config", "Streaming_open", "Streaming_monitor", "Streaming_stop", "Vizualyze", "Form_data_fetch", "Process_analyze", "Start_data_loging", "Pause_data_loging", "Stop_data_loging", "Reset_data_colection", "Error_handler", "Stop"] ("array")
            n320 = local write "Отложенный запуск"(FALSE ("Отложенный запуск")) -> ()
          }
        }
        n321 = case shown="\"2000 л\"" w570 {
          tunnel: w571 -> [w610 w612 w614 w616]
          tunnel: [w609 w611 w613 w615] -> w560
          frame "30 л", Default {
            n322 = Unbundle By Name(w610) -> ("MBA_ch 4"=w609:dbl)
          }
          frame "80 л" {
            n323 = Unbundle By Name(w612) -> ("MBA_ch 1"=w611:dbl)
          }
          frame "800 л" {
            n324 = Unbundle By Name(w614) -> ("MBA_ch 5"=w613:dbl)
          }
          frame "2000 л" {
            n325 = Unbundle By Name(w616) -> ("MBA_ch 8"=w615:dbl)
          }
        }
        "Electrolyte temperature" <- w560
        n326 = call "A-K separation.vi"("Input wave"=w584) -> ("Katod wave (inverted)"=w576:waveform(dbl), "Anod wave"=w577:waveform(dbl))  [unwired: 3 in]
        n327 = call "Termometr_color.vi"("Temperature"=w560) -> ("Scale color"=w559:u32)  [unwired: 8 in]
        n328 = Unbundle By Name(w577) -> ("Y"=w575:dbl[])
        n329 = Unbundle By Name(w576) -> ("Y"=w573:dbl[])
        n330 = property on="Electrolyte temperature" class="Slide (strict)"("Fill Color"=w559) -> ()  [unwired: 2 in, 2 out]
        n331 = Array Max & Min(array=w575) -> (max value=w574:dbl)  [unwired: 3 out]
        n332 = call-poly <vilib>:"RMS.vi"("X"=w575) -> ("rms value"=w597:dbl)  [unwired: 1 out]
        n333 = call-poly <vilib>:"Mean.vi"("X"=w575) -> ("mean"=w598:dbl)  [unwired: 1 out]
        n334 = Array Max & Min(array=w573) -> (max value=w572:dbl)  [unwired: 3 out]
        n335 = call-poly <vilib>:"RMS.vi"("X"=w573) -> ("rms value"=w599:dbl)  [unwired: 1 out]
        n336 = call-poly <vilib>:"Mean.vi"("X"=w573) -> ("mean"=w600:dbl)  [unwired: 1 out]
        n337 = Build Array (concatenate)(w588, w586) -> (w587:T2[])
        n338 = Bundle(w574, "rms value"=w597, "mean"=w598) -> (→"Анодный ток, А":cluster{dbl, "rms value":dbl, "mean":dbl})  [unwired: 1 in]
        n339 = Bundle(w572, "rms value"=w599, "mean"=w600) -> (→"Катодный ток, А":cluster{dbl, "rms value":dbl, "mean":dbl})  [unwired: 1 in]
      }
      frame "Form_data_fetch" {
        w627 = i16 1 ("width (-)")
        # "Амплитудное\nДействующее\nСреднее"
        n340 = Unbundle By Name(w621) -> ("Data log path"=w625:path, "Process_time"=w640:u32)
        n341 = local read "Electrolyte temperature"() -> (w633:dbl)
        n342 = local read "Катодное напряжение, В"() -> (w638:cluster{u16, u16, u16})
        n343 = local read "Анодное напряжение, В"() -> (w637:cluster{u16, u16, u16})
        "Формовочное напряжение" <- w637
        n344 = Divide(x=w640, y=u32 60000) -> (x/y=w636:dbl)
        n345 = local read "Катодный ток, А"() -> (w628:cluster{dbl, dbl, dbl})
        n346 = local read "Анодный ток, А"() -> (w630:cluster{dbl, dbl, dbl})
        "Формовочный ток" <- w630
        n347 = Number To Fractional String(number=w633, precision (6)=i16 1 ("width (-)")) -> (F-format string=w632:string)  [unwired: 2 in]
        n348 = Number To Fractional String(number=w636, precision (6)=i16 1 ("width (-)")) -> (F-format string=w634:string)  [unwired: 2 in]
        n349 = Concatenate Strings(w634, " мин" ("string")) -> (w622:string)
        n350 = Number To Fractional String(number=w630, precision (6)=w627) -> (F-format string=w629:cluster{string, string, string})  [unwired: 2 in]
        n351 = Number To Fractional String(number=w628, precision (6)=w627) -> (F-format string=w626:cluster{string, string, string})  [unwired: 2 in]
        n352 = Number To Decimal String(number=w637) -> (decimal integer string=w658:cluster{string, string, string})  [unwired: 1 in]
        n353 = Number To Decimal String(number=w638) -> (decimal integer string=w639:cluster{string, string, string})  [unwired: 1 in]
        n354 = local read "Voltage"() -> (w624:dbl[])
        n355 = local read "Currency"() -> (w623:dbl[])
        n356 = Unbundle(w658) -> (w649:string, w653:string, w657:string)
        n357 = Unbundle(w639) -> (w647:string, w651:string, w655:string)
        n358 = Unbundle(w629) -> (w648:string, w652:string, w656:string)
        n359 = Unbundle(w626) -> (w646:string, w650:string, w654:string)
        n360 = local read "Process Electrical Parameters"() -> (w645:string[][])
        n361 = call "Write_Temp_Data_Log.vi"("Process_time"=w622, "Current (A)"=w623, "Voltage (V)"=w624, "datalog path (use dialog)"=w625) -> ("error out"=w620:errorcluster)  [unwired: 7 in]
        n362 = Build Array(w622, w657, w656, w655, w654, w653, w652, w651, w650, w649, w648, w647, w646, w632) -> (w644:string[])
        n363 = call <vilib>:"Simple Error Handler.vi"("error in (no error)"=w620) -> ()  [unwired: 4 in, 5 out]
        n364 = Build Array (concatenate)(w645, w644) -> (→"Process Electrical Parameters":string[][])
      }
      frame "Process_analyze" {
        w677 = 20  # i
        # "Усреднение значения на основе i измерений"
        # "Амплитудное\nДействующее \nСреднее"
        n365 = local read "Анодное напряжение, В"() -> (w679:cluster{u16, u16, u16})
        n366 = Unbundle By Name(w661) -> ("Data_write_enable"=w660:bool)
        n367 = Unbundle(w679) -> (w673:u16)  [unwired: 2 out]
        n368 = local read "Max_voltage"() -> (w671:dbl)
        n369 = feedback #13(u16[] []) -> (w676:u16[])
        n370 = Build Array (concatenate)(w676, w673) -> (w678:u16[])
        n371 = Delete From Array(array=w678, length=w677) -> (deleted portion=w674:u16[])  [unwired: 1 in, 1 out]
        n372 = feedback-in #13(w674) -> ()
        n373 = call-poly <vilib>:"Mean.vi"("X"=w674) -> ("mean"=w666:dbl)  [unwired: 1 out]
        n374 = Multiply(x=w671, y=0.9) -> (x*y=w669:dbl)
        n375 = Greater?(x=w673, y=w666) -> (0:w672:bool)
        n376 = Less?(x=w666, y=w669) -> (x < y?=w668:bool)
        n377 = case shown="True" w672 {
          tunnel: w666 -> [_ w705]
          frame False {
          }
          frame True {
            "Max_voltage" <- w705
          }
        }
        n378 = case shown="True" w660 {
          tunnel: w668 -> [_ w688]
          tunnel: [w681 w687] -> w667
          tunnel: w666 -> [_ w686]
          tunnel: [w681 w685] -> w665
          tunnel: [w681 w684] -> w664
          tunnel: [w681 w683] -> w663
          tunnel: [w681 w682] -> w662
          frame False {
            w681 = 3158064  # Темно-серый
          }
          frame True {
            n379 = case shown="False" w688 {
              tunnel: [w702 w704] -> w687
              tunnel: [w701 w703] -> w682
              tunnel: [w700 w703] -> w683
              tunnel: [w699 w703] -> w684
              tunnel: [w698 w703] -> w685
              tunnel: w686 -> [w692 _]
              frame False {
                w690 = 400.0 ("upper limit")
                w689 = 600.0 ("upper limit")
                w693 = 800.0 ("upper limit")
                w697 = 522252  # Зеленый
                w702 = 3158064  # Темно-серый
                n380 = Greater?(x=w692, y=w693) -> (0:w694:bool)
                n381 = Less?(x=w692, y=w690) -> (x < y?=w691:bool)
                n382 = In Range and Coerce(upper limit=w693, x=w692, lower limit=w689) -> (In Range?=w696:bool)  [unwired: 1 out]
                n383 = In Range and Coerce(upper limit=w689, x=w692, lower limit=w690) -> (In Range?=w695:bool)  [unwired: 1 out]
                n384 = Select(t=w697, s=w694, f=w702) -> (s? t:f=w701:i32)
                n385 = Select(t=w697, s=w696, f=w702) -> (s? t:f=w700:i32)
                n386 = Select(t=w697, s=w695, f=w702) -> (s? t:f=w699:i32)
                n387 = Select(t=w697, s=w691, f=w702) -> (s? t:f=w698:i32)
              }
              frame True {
                w703 = 3158064  # Темно-серый
                w704 = 16254993  # Красный
                # "Угасание"
              }
            }
          }
        }
        n388 = property on="ДР" class="Str"("Text.BGColor"=w662) -> ()  [unwired: 2 in, 2 out]
        n389 = property on="МДР" class="Str"("Text.BGColor"=w663) -> ()  [unwired: 2 in, 2 out]
        n390 = property on="ИР" class="Str"("Text.BGColor"=w664) -> ()  [unwired: 2 in, 2 out]
        n391 = property on="ГАЛЬВ.ЛЮМ." class="Str"("Text.BGColor"=w665) -> ()  [unwired: 2 in, 2 out]
        n392 = property on="УГАСАНИЕ" class="Str"("Text.BGColor"=w667) -> ()  [unwired: 2 in, 2 out]
      }
      frame "Start_data_loging" {
        n393 = in-place {
          w710 = 522252  # Зеленый
          w715 = 3158064  # Темно-серый
          n394 = in-place-cluster #14(w707) -> ("Streaming_enable"=w716:bool)  [unwired: 2 out]
          n395 = case shown="True" w716 {
            tunnel: w715 -> [w717 w718]
            tunnel: [w717 w718] -> w714
            tunnel: [w717 w719] -> w713
            tunnel: [w717 w718] -> w712
            tunnel: [w717 w718] -> w711
            tunnel: w710 -> [_ w719]
            frame False {
            }
            frame True {
            }
          }
          n396 = property on="Готовность" class="Str"("Text.BGColor"=w714) -> ()  [unwired: 2 in, 2 out]
          n397 = property on="СБОР" class="Str"("Text.BGColor"=w713) -> ()  [unwired: 2 in, 2 out]
          n398 = property on="ПАУЗА" class="Str"("Text.BGColor"=w712) -> ()  [unwired: 2 in, 2 out]
          n399 = property on="СТОП" class="Str"("Text.BGColor"=w711) -> ()  [unwired: 2 in, 2 out]
          n400 = Tick Count (ms)() -> (millisecond timer value=w709:u32)
          n401 = in-place-cluster #14("Streaming_enable"=w716, "Data_write_enable"=w716, "startup_time"=w709) -> (w706:T6)
        }
      }
      frame "Pause_data_loging" {
        n402 = in-place {
          w725 = 15989767  # Желтый
          w730 = 522252  # Зеленый
          w731 = 3158064  # Темно-серый
          n403 = in-place-cluster #15(w722) -> ("Streaming_enable"=w732:bool)  [unwired: 1 out]
          n404 = case shown="False" "Пауза" {
            tunnel: w731 -> [w734 w737]
            tunnel: [w734 w737] -> w729
            tunnel: [w734 w737] -> w728
            tunnel: [w734 w736] -> w727
            tunnel: [w734 w737] -> w726
            tunnel: w730 -> [_ _]
            tunnel: w725 -> [_ w736]
            tunnel: [TRUE ("Data_write_enable") FALSE ("Data_write_enable")] -> w724
            frame False {
            }
            frame True {
            }
          }
          n405 = property on="Готовность" class="Str"("Text.BGColor"=w729) -> ()  [unwired: 2 in, 2 out]
          n406 = property on="СБОР" class="Str"("Text.BGColor"=w728) -> ()  [unwired: 2 in, 2 out]
          n407 = property on="ПАУЗА" class="Str"("Text.BGColor"=w727) -> ()  [unwired: 2 in, 2 out]
          n408 = property on="СТОП" class="Str"("Text.BGColor"=w726) -> ()  [unwired: 2 in, 2 out]
          n409 = in-place-cluster #15("Streaming_enable"=w732, "Data_write_enable"=w724) -> (w721:T6)
        }
      }
      frame "Stop_data_loging" {
        n410 = in-place {
          w741 = 16254993  # Красный
          w748 = 522252  # Зеленый
          w749 = 3158064  # Темно-серый
          n411 = in-place-cluster #16(w740) -> ("Streaming_enable"=w750:bool)  [unwired: 2 out]
          n412 = case shown="True" w750 {
            tunnel: w749 -> [w751 w753]
            tunnel: [w751 w753] -> w746
            tunnel: [w751 w753] -> w745
            tunnel: [w751 w753] -> w744
            tunnel: [w751 w752] -> w743
            tunnel: w748 -> [_ _]
            tunnel: w741 -> [_ w752]
            frame False {
            }
            frame True {
            }
          }
          n413 = property on="Готовность" class="Str"("Text.BGColor"=w746) -> ()  [unwired: 2 in, 2 out]
          n414 = property on="СБОР" class="Str"("Text.BGColor"=w745) -> ()  [unwired: 2 in, 2 out]
          n415 = property on="ПАУЗА" class="Str"("Text.BGColor"=w744) -> ()  [unwired: 2 in, 2 out]
          n416 = property on="СТОП" class="Str"("Text.BGColor"=w743) -> ()  [unwired: 2 in, 2 out]
          n417 = in-place-cluster #16("Streaming_enable"=w750, "Data_write_enable"=FALSE, "startup_time"=u32 0) -> (w739:T6)
        }
      }
      frame "Reset_data_colection" {
        w761 = 3158064  # Темно-серый
        w763 = cluster{u16, u16, u16}[] [] ("History Data")
        n418 = Unbundle By Name(w755) -> ("Data log path"=w754:path)
        n419 = property on="Формовочное напряжение" class="WFChart (strict)"("History Data"=w763) -> ()  [unwired: 2 in, 2 out]
        n420 = property on="Формовочный ток" class="WFChart (strict)"("History Data"=w763) -> ()  [unwired: 2 in, 2 out]
        n421 = local write "Process Electrical Parameters"(string[][] [] ("Process Electrical Parameters")) -> ()
        n422 = Open/Create/Replace Datalog(5:cluster{string, "empty array":sgl[]} {"", "empty array"=[]}, 10:T11."replace" ("operation (0:open)"), 11:w754) -> (0:w757:errorcluster, 3:w756:refnum<k1>)  [unwired: 1 in, 3 out]
        n423 = Close File(refnum=w756, error in=w757) -> ()  [unwired: 2 out]
        n424 = local write "Max_voltage"(0.0 ("Max_voltage")) -> ()
        n425 = property on="ДАННЫЕ СОХРАНЕНЫ" class="Str"("Text.BGColor"=w761) -> ()  [unwired: 2 in, 2 out]
      }
      frame "Error_handler" {
        n426 = in-place {
          in-place-border: w766 -> [w775]
          in-place-border: [w774] -> w765
          w773 = T2[] [enum."Streaming_stop", enum."Streaming_config", enum."Streaming_open"] items=["Wait_for_event", "Initialize", "Save_ini", "Save_data", "Streaming_config", "Streaming_open", "Streaming_monitor", "Streaming_stop", "Vizualyze", "Form_data_fetch", "Process_analyze", "Start_data_loging", "Pause_data_loging", "Stop_data_loging", "Reset_data_colection", "Error_handler", "Stop"] ("array")
          n427 = in-place-cluster #17(w768) -> ("Global_errors"=w769:errorcluster)
          n428 = feedback-in #18(w769) -> ()
          n429 = feedback #18(errorcluster {"status"=FALSE, "code"=0, "source"=""} ("Global_errors")) -> (w771:errorcluster)
          n430 = Equal?(x=w769, y=w771) -> (x = y?=w770:bool)
          n431 = case shown="False" w770 {
            tunnel: w769 -> [w778 _]
            frame False {
              w777 = T13 3 items=["no dialog", "OK message", "continue or stop message", "OK message + warnings", "continue/stop + warnings"] ("type of dialog (OK msg:1)")
              n432 = call <vilib>:"General Error Handler.vi"("type of dialog (OK msg:1)"=w777, "error in (no error)"=w778) -> ()  [unwired: 9 in, 5 out]
            }
            frame True {
            }
          }
          n433 = Build Array (concatenate)(w775, w773) -> (w774:T2[])
          n434 = in-place-cluster #17("Global_errors"=errorcluster {"status"=FALSE, "code"=0, "source"=""}) -> (w767:T6)
        }
      }
      frame "Stop" {
      }
    }
    n435 = Equal?(x=w8, y=main_states."Stop") -> (x = y?=w23:bool)
    n436 = property on="current_state" class="Enum (strict)"() -> ("RingText.Text"=w20:string)  [unwired: 2 in, 2 out]
    n437 = feedback #19("") -> (w11:string)
    n438 = Concatenate Strings(w20, "\r", w11) -> (w21:string)
    n439 = String Subset(string=w21, length (rest)=1000 ("length (rest)")) -> (substring=w17:string)  [unwired: 1 in]
    "states_history" <- w17
    n440 = feedback-in #19(w17) -> ()
  }
  n441 = Unbundle By Name(w5) -> ("shutdown?"=w1:bool)
  n442 = property class="App"() -> (reference out=w4:refnum<vi>, error out=w3:errorcluster, "App.Kind"=w2:T12)  [unwired: 2 in]
  n443 = Close Reference(reference=w4, error in (no error)=w3) -> ()  [unwired: 1 out]
  n444 = case shown="\"Run Time System\"" w2 {
    tunnel: w1 -> [_ w781]
    frame "Development System", Default {
    }
    frame "Run Time System" {
      n445 = stacked-sequence {
        tunnel: w781 -> [w782 _]
        frame #0 {
          n446 = case shown="True" w782 {
            frame False {
            }
            frame True {
              n447 = call <vilib>:"System Exec.vi"("command line"="Shutdown /s /t 0") -> ()  [unwired: 7 in, 4 out]
            }
          }
        }
        frame #1 {
          n448 = Quit LabVIEW(quit? (T)=TRUE) -> ()
        }
      }
    }
  }
